vi "GetRadialProfile2.vi"(0 "Which \nRadial Profile? 2":enum16{"Cold Image", "Hot/Cold", "Hot Image"}(ring)=enum."Hot/Cold" caption="Which Radial Profile?", 1 "Paths in Folder":path[](array[path])=[path "C:/Daten/pHGradienten/130403_Cy5_74mer_TRIS/130403_Cy5_74mer_TRIS/A_50mM_TRIS/50mA/TRIS_50mM_50mA_000001.tif", path "C:/Daten/pHGradienten/130403_Cy5_74mer_TRIS/130403_Cy5_74mer_TRIS/A_50mM_TRIS/50mA/TRIS_50mM_50mA_000002.tif", path "C:/Daten/pHGradienten/130403_Cy5_74mer_TRIS/130403_Cy5_74mer_TRIS/A_50mM_TRIS/50mA/TRIS_50mM_50mA_000003.tif", path "C:/Daten/pHGradienten/130403_Cy5_74mer_TRIS/130403_Cy5_74mer_TRIS/A_50mM_TRIS/50mA/TRIS_50mM_50mA_000004.tif", path "C:/Daten/pHGradienten/130403_Cy5_74mer_TRIS/130403_Cy5_74mer_TRIS/A_50mM_TRIS/50mA/TRIS_50mM_50mA_000005.tif", path "C:/Daten/pHGradienten/130403_Cy5_74mer_TRIS/130403_Cy5_74mer_TRIS/A_50mM_TRIS/50mA/TRIS_50mM_50mA_000006.tif", path "C:/Daten/pHGradienten/130403_Cy5_74mer_TRIS/130403_Cy5_74mer_TRIS/A_50mM_TRIS/50mA/TRIS_50mM_50mA_000007.tif", path "C:/Daten/pHGradienten/130403_Cy5_74mer_TRIS/130403_Cy5_74mer_TRIS/A_50mM_TRIS/50mA/TRIS_50mM_50mA_000008.tif", path "C:/Daten/pHGradienten/130403_Cy5_74mer_TRIS/130403_Cy5_74mer_TRIS/A_50mM_TRIS/50mA/TRIS_50mM_50mA_000009.tif", path "C:/Daten/pHGradienten/130403_Cy5_74mer_TRIS/130403_Cy5_74mer_TRIS/A_50mM_TRIS/50mA/TRIS_50mM_50mA_000010.tif", path "C:/Daten/pHGradienten/130403_Cy5_74mer_TRIS/130403_Cy5_74mer_TRIS/A_50mM_TRIS/50mA/TRIS_50mM_50mA_000011.tif", path "C:/Daten/pHGradienten/130403_Cy5_74mer_TRIS/130403_Cy5_74mer_TRIS/A_50mM_TRIS/50mA/TRIS_50mM_50mA_000012.tif", path "C:/Daten/pHGradienten/130403_Cy5_74mer_TRIS/130403_Cy5_74mer_TRIS/A_50mM_TRIS/50mA/TRIS_50mM_50mA_000013.tif", path "C:/Daten/pHGradienten/130403_Cy5_74mer_TRIS/130403_Cy5_74mer_TRIS/A_50mM_TRIS/50mA/TRIS_50mM_50mA_000014.tif", path "C:/Daten/pHGradienten/130403_Cy5_74mer_TRIS/130403_Cy5_74mer_TRIS/A_50mM_TRIS/50mA/TRIS_50mM_50mA_000015.tif", path "C:/Daten/pHGradienten/130403_Cy5_74mer_TRIS/130403_Cy5_74mer_TRIS/A_50mM_TRIS/50mA/TRIS_50mM_50mA_000016.tif", path "C:/Daten/pHGradienten/130403_Cy5_74mer_TRIS/130403_Cy5_74mer_TRIS/A_50mM_TRIS/50mA/TRIS_50mM_50mA_000017.tif", path "C:/Daten/pHGradienten/130403_Cy5_74mer_TRIS/130403_Cy5_74mer_TRIS/A_50mM_TRIS/50mA/TRIS_50mM_50mA_000018.tif", path "C:/Daten/pHGradienten/130403_Cy5_74mer_TRIS/130403_Cy5_74mer_TRIS/A_50mM_TRIS/50mA/TRIS_50mM_50mA_000019.tif", path "C:/Daten/pHGradienten/130403_Cy5_74mer_TRIS/130403_Cy5_74mer_TRIS/A_50mM_TRIS/50mA/TRIS_50mM_50mA_000020.tif", path "C:/Daten/pHGradienten/130403_Cy5_74mer_TRIS/130403_Cy5_74mer_TRIS/A_50mM_TRIS/50mA/TRIS_50mM_50mA_000021.tif", path "C:/Daten/pHGradienten/130403_Cy5_74mer_TRIS/130403_Cy5_74mer_TRIS/A_50mM_TRIS/50mA/TRIS_50mM_50mA_000022.tif", path "C:/Daten/pHGradienten/130403_Cy5_74mer_TRIS/130403_Cy5_74mer_TRIS/A_50mM_TRIS/50mA/TRIS_50mM_50mA_000023.tif", path "C:/Daten/pHGradienten/130403_Cy5_74mer_TRIS/130403_Cy5_74mer_TRIS/A_50mM_TRIS/50mA/TRIS_50mM_50mA_000024.tif", path "C:/Daten/pHGradienten/130403_Cy5_74mer_TRIS/130403_Cy5_74mer_TRIS/A_50mM_TRIS/50mA/TRIS_50mM_50mA_000025.tif", path "C:/Daten/pHGradienten/130403_Cy5_74mer_TRIS/130403_Cy5_74mer_TRIS/A_50mM_TRIS/50mA/TRIS_50mM_50mA_000026.tif", path "C:/Daten/pHGradienten/130403_Cy5_74mer_TRIS/130403_Cy5_74mer_TRIS/A_50mM_TRIS/50mA/TRIS_50mM_50mA_000027.tif", path "C:/Daten/pHGradienten/130403_Cy5_74mer_TRIS/130403_Cy5_74mer_TRIS/A_50mM_TRIS/50mA/TRIS_50mM_50mA_000028.tif", path "C:/Daten/pHGradienten/130403_Cy5_74mer_TRIS/130403_Cy5_74mer_TRIS/A_50mM_TRIS/50mA/TRIS_50mM_50mA_000029.tif", path "C:/Daten/pHGradienten/130403_Cy5_74mer_TRIS/130403_Cy5_74mer_TRIS/A_50mM_TRIS/50mA/TRIS_50mM_50mA_000030.tif", path "C:/Daten/pHGradienten/130403_Cy5_74mer_TRIS/130403_Cy5_74mer_TRIS/A_50mM_TRIS/50mA/TRIS_50mM_50mA_000031.tif", path "C:/Daten/pHGradienten/130403_Cy5_74mer_TRIS/130403_Cy5_74mer_TRIS/A_50mM_TRIS/50mA/TRIS_50mM_50mA_000032.tif", path "C:/Daten/pHGradienten/130403_Cy5_74mer_TRIS/130403_Cy5_74mer_TRIS/A_50mM_TRIS/50mA/TRIS_50mM_50mA_000033.tif", path "C:/Daten/pHGradienten/130403_Cy5_74mer_TRIS/130403_Cy5_74mer_TRIS/A_50mM_TRIS/50mA/TRIS_50mM_50mA_000034.tif", path "C:/Daten/pHGradienten/130403_Cy5_74mer_TRIS/130403_Cy5_74mer_TRIS/A_50mM_TRIS/50mA/TRIS_50mM_50mA_000035.tif", path "C:/Daten/pHGradienten/130403_Cy5_74mer_TRIS/130403_Cy5_74mer_TRIS/A_50mM_TRIS/50mA/TRIS_50mM_50mA_000036.tif", path "C:/Daten/pHGradienten/130403_Cy5_74mer_TRIS/130403_Cy5_74mer_TRIS/A_50mM_TRIS/50mA/TRIS_50mM_50mA_000037.tif", path "C:/Daten/pHGradienten/130403_Cy5_74mer_TRIS/130403_Cy5_74mer_TRIS/A_50mM_TRIS/50mA/TRIS_50mM_50mA_000038.tif", path "C:/Daten/pHGradienten/130403_Cy5_74mer_TRIS/130403_Cy5_74mer_TRIS/A_50mM_TRIS/50mA/TRIS_50mM_50mA_000039.tif", path "C:/Daten/pHGradienten/130403_Cy5_74mer_TRIS/130403_Cy5_74mer_TRIS/A_50mM_TRIS/50mA/TRIS_50mM_50mA_000040.tif", path "C:/Daten/pHGradienten/130403_Cy5_74mer_TRIS/130403_Cy5_74mer_TRIS/A_50mM_TRIS/50mA/TRIS_50mM_50mA_000041.tif", path "C:/Daten/pHGradienten/130403_Cy5_74mer_TRIS/130403_Cy5_74mer_TRIS/A_50mM_TRIS/50mA/TRIS_50mM_50mA_000042.tif", path "C:/Daten/pHGradienten/130403_Cy5_74mer_TRIS/130403_Cy5_74mer_TRIS/A_50mM_TRIS/50mA/TRIS_50mM_50mA_000043.tif", path "C:/Daten/pHGradienten/130403_Cy5_74mer_TRIS/130403_Cy5_74mer_TRIS/A_50mM_TRIS/50mA/TRIS_50mM_50mA_000044.tif", path "C:/Daten/pHGradienten/130403_Cy5_74mer_TRIS/130403_Cy5_74mer_TRIS/A_50mM_TRIS/50mA/TRIS_50mM_50mA_000045.tif", path "C:/Daten/pHGradienten/130403_Cy5_74mer_TRIS/130403_Cy5_74mer_TRIS/A_50mM_TRIS/50mA/TRIS_50mM_50mA_000046.tif", path "C:/Daten/pHGradienten/130403_Cy5_74mer_TRIS/130403_Cy5_74mer_TRIS/A_50mM_TRIS/50mA/TRIS_50mM_50mA_000047.tif", path "C:/Daten/pHGradienten/130403_Cy5_74mer_TRIS/130403_Cy5_74mer_TRIS/A_50mM_TRIS/50mA/TRIS_50mM_50mA_000048.tif", path "C:/Daten/pHGradienten/130403_Cy5_74mer_TRIS/130403_Cy5_74mer_TRIS/A_50mM_TRIS/50mA/TRIS_50mM_50mA_000049.tif", path "C:/Daten/pHGradienten/130403_Cy5_74mer_TRIS/130403_Cy5_74mer_TRIS/A_50mM_TRIS/50mA/TRIS_50mM_50mA_000050.tif", path "C:/Daten/pHGradienten/130403_Cy5_74mer_TRIS/130403_Cy5_74mer_TRIS/A_50mM_TRIS/50mA/TRIS_50mM_50mA_000051.tif", path "C:/Daten/pHGradienten/130403_Cy5_74mer_TRIS/130403_Cy5_74mer_TRIS/A_50mM_TRIS/50mA/TRIS_50mM_50mA_000052.tif", path "C:/Daten/pHGradienten/130403_Cy5_74mer_TRIS/130403_Cy5_74mer_TRIS/A_50mM_TRIS/50mA/TRIS_50mM_50mA_000053.tif", path "C:/Daten/pHGradienten/130403_Cy5_74mer_TRIS/130403_Cy5_74mer_TRIS/A_50mM_TRIS/50mA/TRIS_50mM_50mA_000054.tif", path "C:/Daten/pHGradienten/130403_Cy5_74mer_TRIS/130403_Cy5_74mer_TRIS/A_50mM_TRIS/50mA/TRIS_50mM_50mA_000055.tif", path "C:/Daten/pHGradienten/130403_Cy5_74mer_TRIS/130403_Cy5_74mer_TRIS/A_50mM_TRIS/50mA/TRIS_50mM_50mA_000056.tif", path "C:/Daten/pHGradienten/130403_Cy5_74mer_TRIS/130403_Cy5_74mer_TRIS/A_50mM_TRIS/50mA/TRIS_50mM_50mA_000057.tif", path "C:/Daten/pHGradienten/130403_Cy5_74mer_TRIS/130403_Cy5_74mer_TRIS/A_50mM_TRIS/50mA/TRIS_50mM_50mA_000058.tif", path "C:/Daten/pHGradienten/130403_Cy5_74mer_TRIS/130403_Cy5_74mer_TRIS/A_50mM_TRIS/50mA/TRIS_50mM_50mA_000059.tif", path "C:/Daten/pHGradienten/130403_Cy5_74mer_TRIS/130403_Cy5_74mer_TRIS/A_50mM_TRIS/50mA/TRIS_50mM_50mA_000060.tif", path "C:/Daten/pHGradienten/130403_Cy5_74mer_TRIS/130403_Cy5_74mer_TRIS/A_50mM_TRIS/50mA/TRIS_50mM_50mA_000061.tif", path "C:/Daten/pHGradienten/130403_Cy5_74mer_TRIS/130403_Cy5_74mer_TRIS/A_50mM_TRIS/50mA/TRIS_50mM_50mA_000062.tif", path "C:/Daten/pHGradienten/130403_Cy5_74mer_TRIS/130403_Cy5_74mer_TRIS/A_50mM_TRIS/50mA/TRIS_50mM_50mA_000063.tif", path "C:/Daten/pHGradienten/130403_Cy5_74mer_TRIS/130403_Cy5_74mer_TRIS/A_50mM_TRIS/50mA/TRIS_50mM_50mA_000064.tif", path "C:/Daten/pHGradienten/130403_Cy5_74mer_TRIS/130403_Cy5_74mer_TRIS/A_50mM_TRIS/50mA/TRIS_50mM_50mA_000065.tif", path "C:/Daten/pHGradienten/130403_Cy5_74mer_TRIS/130403_Cy5_74mer_TRIS/A_50mM_TRIS/50mA/TRIS_50mM_50mA_000066.tif", path "C:/Daten/pHGradienten/130403_Cy5_74mer_TRIS/130403_Cy5_74mer_TRIS/A_50mM_TRIS/50mA/TRIS_50mM_50mA_000067.tif", path "C:/Daten/pHGradienten/130403_Cy5_74mer_TRIS/130403_Cy5_74mer_TRIS/A_50mM_TRIS/50mA/TRIS_50mM_50mA_000068.tif", path "C:/Daten/pHGradienten/130403_Cy5_74mer_TRIS/130403_Cy5_74mer_TRIS/A_50mM_TRIS/50mA/TRIS_50mM_50mA_000069.tif", path "C:/Daten/pHGradienten/130403_Cy5_74mer_TRIS/130403_Cy5_74mer_TRIS/A_50mM_TRIS/50mA/TRIS_50mM_50mA_000070.tif", path "C:/Daten/pHGradienten/130403_Cy5_74mer_TRIS/130403_Cy5_74mer_TRIS/A_50mM_TRIS/50mA/TRIS_50mM_50mA_000071.tif", path "C:/Daten/pHGradienten/130403_Cy5_74mer_TRIS/130403_Cy5_74mer_TRIS/A_50mM_TRIS/50mA/TRIS_50mM_50mA_000072.tif", path "C:/Daten/pHGradienten/130403_Cy5_74mer_TRIS/130403_Cy5_74mer_TRIS/A_50mM_TRIS/50mA/TRIS_50mM_50mA_000073.tif", path "C:/Daten/pHGradienten/130403_Cy5_74mer_TRIS/130403_Cy5_74mer_TRIS/A_50mM_TRIS/50mA/TRIS_50mM_50mA_000074.tif", path "C:/Daten/pHGradienten/130403_Cy5_74mer_TRIS/130403_Cy5_74mer_TRIS/A_50mM_TRIS/50mA/TRIS_50mM_50mA_000075.tif", path "C:/Daten/pHGradienten/130403_Cy5_74mer_TRIS/130403_Cy5_74mer_TRIS/A_50mM_TRIS/50mA/TRIS_50mM_50mA_000076.tif", path "C:/Daten/pHGradienten/130403_Cy5_74mer_TRIS/130403_Cy5_74mer_TRIS/A_50mM_TRIS/50mA/TRIS_50mM_50mA_000077.tif", path "C:/Daten/pHGradienten/130403_Cy5_74mer_TRIS/130403_Cy5_74mer_TRIS/A_50mM_TRIS/50mA/TRIS_50mM_50mA_000078.tif", path "C:/Daten/pHGradienten/130403_Cy5_74mer_TRIS/130403_Cy5_74mer_TRIS/A_50mM_TRIS/50mA/TRIS_50mM_50mA_000079.tif", path "C:/Daten/pHGradienten/130403_Cy5_74mer_TRIS/130403_Cy5_74mer_TRIS/A_50mM_TRIS/50mA/TRIS_50mM_50mA_000080.tif", path "C:/Daten/pHGradienten/130403_Cy5_74mer_TRIS/130403_Cy5_74mer_TRIS/A_50mM_TRIS/50mA/TRIS_50mM_50mA_000081.tif", path "C:/Daten/pHGradienten/130403_Cy5_74mer_TRIS/130403_Cy5_74mer_TRIS/A_50mM_TRIS/50mA/TRIS_50mM_50mA_000082.tif", path "C:/Daten/pHGradienten/130403_Cy5_74mer_TRIS/130403_Cy5_74mer_TRIS/A_50mM_TRIS/50mA/TRIS_50mM_50mA_000083.tif", path "C:/Daten/pHGradienten/130403_Cy5_74mer_TRIS/130403_Cy5_74mer_TRIS/A_50mM_TRIS/50mA/TRIS_50mM_50mA_000084.tif", path "C:/Daten/pHGradienten/130403_Cy5_74mer_TRIS/130403_Cy5_74mer_TRIS/A_50mM_TRIS/50mA/TRIS_50mM_50mA_000085.tif", path "C:/Daten/pHGradienten/130403_Cy5_74mer_TRIS/130403_Cy5_74mer_TRIS/A_50mM_TRIS/50mA/TRIS_50mM_50mA_000086.tif", path "C:/Daten/pHGradienten/130403_Cy5_74mer_TRIS/130403_Cy5_74mer_TRIS/A_50mM_TRIS/50mA/TRIS_50mM_50mA_000087.tif", path "C:/Daten/pHGradienten/130403_Cy5_74mer_TRIS/130403_Cy5_74mer_TRIS/A_50mM_TRIS/50mA/TRIS_50mM_50mA_000088.tif", path "C:/Daten/pHGradienten/130403_Cy5_74mer_TRIS/130403_Cy5_74mer_TRIS/A_50mM_TRIS/50mA/TRIS_50mM_50mA_000089.tif", path "C:/Daten/pHGradienten/130403_Cy5_74mer_TRIS/130403_Cy5_74mer_TRIS/A_50mM_TRIS/50mA/TRIS_50mM_50mA_000090.tif", path "C:/Daten/pHGradienten/130403_Cy5_74mer_TRIS/130403_Cy5_74mer_TRIS/A_50mM_TRIS/50mA/TRIS_50mM_50mA_000091.tif", path "C:/Daten/pHGradienten/130403_Cy5_74mer_TRIS/130403_Cy5_74mer_TRIS/A_50mM_TRIS/50mA/TRIS_50mM_50mA_000092.tif", path "C:/Daten/pHGradienten/130403_Cy5_74mer_TRIS/130403_Cy5_74mer_TRIS/A_50mM_TRIS/50mA/TRIS_50mM_50mA_000093.tif", path "C:/Daten/pHGradienten/130403_Cy5_74mer_TRIS/130403_Cy5_74mer_TRIS/A_50mM_TRIS/50mA/TRIS_50mM_50mA_000094.tif", path "C:/Daten/pHGradienten/130403_Cy5_74mer_TRIS/130403_Cy5_74mer_TRIS/A_50mM_TRIS/50mA/TRIS_50mM_50mA_000095.tif", path "C:/Daten/pHGradienten/130403_Cy5_74mer_TRIS/130403_Cy5_74mer_TRIS/A_50mM_TRIS/50mA/TRIS_50mM_50mA_000096.tif", path "C:/Daten/pHGradienten/130403_Cy5_74mer_TRIS/130403_Cy5_74mer_TRIS/A_50mM_TRIS/50mA/TRIS_50mM_50mA_000097.tif", path "C:/Daten/pHGradienten/130403_Cy5_74mer_TRIS/130403_Cy5_74mer_TRIS/A_50mM_TRIS/50mA/TRIS_50mM_50mA_000098.tif", path "C:/Daten/pHGradienten/130403_Cy5_74mer_TRIS/130403_Cy5_74mer_TRIS/A_50mM_TRIS/50mA/TRIS_50mM_50mA_000099.tif", path "C:/Daten/pHGradienten/130403_Cy5_74mer_TRIS/130403_Cy5_74mer_TRIS/A_50mM_TRIS/50mA/TRIS_50mM_50mA_000100.tif", path "C:/Daten/pHGradienten/130403_Cy5_74mer_TRIS/130403_Cy5_74mer_TRIS/A_50mM_TRIS/50mA/TRIS_50mM_50mA_000101.tif", path "C:/Daten/pHGradienten/130403_Cy5_74mer_TRIS/130403_Cy5_74mer_TRIS/A_50mM_TRIS/50mA/TRIS_50mM_50mA_000102.tif", path "C:/Daten/pHGradienten/130403_Cy5_74mer_TRIS/130403_Cy5_74mer_TRIS/A_50mM_TRIS/50mA/TRIS_50mM_50mA_000103.tif", path "C:/Daten/pHGradienten/130403_Cy5_74mer_TRIS/130403_Cy5_74mer_TRIS/A_50mM_TRIS/50mA/TRIS_50mM_50mA_000104.tif", path "C:/Daten/pHGradienten/130403_Cy5_74mer_TRIS/130403_Cy5_74mer_TRIS/A_50mM_TRIS/50mA/TRIS_50mM_50mA_000105.tif", path "C:/Daten/pHGradienten/130403_Cy5_74mer_TRIS/130403_Cy5_74mer_TRIS/A_50mM_TRIS/50mA/TRIS_50mM_50mA_000106.tif", path "C:/Daten/pHGradienten/130403_Cy5_74mer_TRIS/130403_Cy5_74mer_TRIS/A_50mM_TRIS/50mA/TRIS_50mM_50mA_000107.tif", path "C:/Daten/pHGradienten/130403_Cy5_74mer_TRIS/130403_Cy5_74mer_TRIS/A_50mM_TRIS/50mA/TRIS_50mM_50mA_000108.tif", path "C:/Daten/pHGradienten/130403_Cy5_74mer_TRIS/130403_Cy5_74mer_TRIS/A_50mM_TRIS/50mA/TRIS_50mM_50mA_000109.tif", path "C:/Daten/pHGradienten/130403_Cy5_74mer_TRIS/130403_Cy5_74mer_TRIS/A_50mM_TRIS/50mA/TRIS_50mM_50mA_000110.tif", path "C:/Daten/pHGradienten/130403_Cy5_74mer_TRIS/130403_Cy5_74mer_TRIS/A_50mM_TRIS/50mA/TRIS_50mM_50mA_000111.tif", path "C:/Daten/pHGradienten/130403_Cy5_74mer_TRIS/130403_Cy5_74mer_TRIS/A_50mM_TRIS/50mA/TRIS_50mM_50mA_000112.tif", path "C:/Daten/pHGradienten/130403_Cy5_74mer_TRIS/130403_Cy5_74mer_TRIS/A_50mM_TRIS/50mA/TRIS_50mM_50mA_000113.tif", path "C:/Daten/pHGradienten/130403_Cy5_74mer_TRIS/130403_Cy5_74mer_TRIS/A_50mM_TRIS/50mA/TRIS_50mM_50mA_000114.tif", path "C:/Daten/pHGradienten/130403_Cy5_74mer_TRIS/130403_Cy5_74mer_TRIS/A_50mM_TRIS/50mA/TRIS_50mM_50mA_000115.tif", path "C:/Daten/pHGradienten/130403_Cy5_74mer_TRIS/130403_Cy5_74mer_TRIS/A_50mM_TRIS/50mA/TRIS_50mM_50mA_000116.tif", path "C:/Daten/pHGradienten/130403_Cy5_74mer_TRIS/130403_Cy5_74mer_TRIS/A_50mM_TRIS/50mA/TRIS_50mM_50mA_000117.tif", path "C:/Daten/pHGradienten/130403_Cy5_74mer_TRIS/130403_Cy5_74mer_TRIS/A_50mM_TRIS/50mA/TRIS_50mM_50mA_000118.tif", path "C:/Daten/pHGradienten/130403_Cy5_74mer_TRIS/130403_Cy5_74mer_TRIS/A_50mM_TRIS/50mA/TRIS_50mM_50mA_000119.tif", path "C:/Daten/pHGradienten/130403_Cy5_74mer_TRIS/130403_Cy5_74mer_TRIS/A_50mM_TRIS/50mA/TRIS_50mM_50mA_000120.tif", path "C:/Daten/pHGradienten/130403_Cy5_74mer_TRIS/130403_Cy5_74mer_TRIS/A_50mM_TRIS/50mA/TRIS_50mM_50mA_000121.tif", path "C:/Daten/pHGradienten/130403_Cy5_74mer_TRIS/130403_Cy5_74mer_TRIS/A_50mM_TRIS/50mA/TRIS_50mM_50mA_000122.tif", path "C:/Daten/pHGradienten/130403_Cy5_74mer_TRIS/130403_Cy5_74mer_TRIS/A_50mM_TRIS/50mA/TRIS_50mM_50mA_000123.tif", path "C:/Daten/pHGradienten/130403_Cy5_74mer_TRIS/130403_Cy5_74mer_TRIS/A_50mM_TRIS/50mA/TRIS_50mM_50mA_000124.tif", path "C:/Daten/pHGradienten/130403_Cy5_74mer_TRIS/130403_Cy5_74mer_TRIS/A_50mM_TRIS/50mA/TRIS_50mM_50mA_000125.tif", path "C:/Daten/pHGradienten/130403_Cy5_74mer_TRIS/130403_Cy5_74mer_TRIS/A_50mM_TRIS/50mA/TRIS_50mM_50mA_000126.tif", path "C:/Daten/pHGradienten/130403_Cy5_74mer_TRIS/130403_Cy5_74mer_TRIS/A_50mM_TRIS/50mA/TRIS_50mM_50mA_000127.tif", path "C:/Daten/pHGradienten/130403_Cy5_74mer_TRIS/130403_Cy5_74mer_TRIS/A_50mM_TRIS/50mA/TRIS_50mM_50mA_000128.tif", path "C:/Daten/pHGradienten/130403_Cy5_74mer_TRIS/130403_Cy5_74mer_TRIS/A_50mM_TRIS/50mA/TRIS_50mM_50mA_000129.tif", path "C:/Daten/pHGradienten/130403_Cy5_74mer_TRIS/130403_Cy5_74mer_TRIS/A_50mM_TRIS/50mA/TRIS_50mM_50mA_000130.tif", path "C:/Daten/pHGradienten/130403_Cy5_74mer_TRIS/130403_Cy5_74mer_TRIS/A_50mM_TRIS/50mA/TRIS_50mM_50mA_000131.tif", path "C:/Daten/pHGradienten/130403_Cy5_74mer_TRIS/130403_Cy5_74mer_TRIS/A_50mM_TRIS/50mA/TRIS_50mM_50mA_000132.tif", path "C:/Daten/pHGradienten/130403_Cy5_74mer_TRIS/130403_Cy5_74mer_TRIS/A_50mM_TRIS/50mA/TRIS_50mM_50mA_000133.tif", path "C:/Daten/pHGradienten/130403_Cy5_74mer_TRIS/130403_Cy5_74mer_TRIS/A_50mM_TRIS/50mA/TRIS_50mM_50mA_000134.tif", path "C:/Daten/pHGradienten/130403_Cy5_74mer_TRIS/130403_Cy5_74mer_TRIS/A_50mM_TRIS/50mA/TRIS_50mM_50mA_000135.tif", path "C:/Daten/pHGradienten/130403_Cy5_74mer_TRIS/130403_Cy5_74mer_TRIS/A_50mM_TRIS/50mA/TRIS_50mM_50mA_000136.tif", path "C:/Daten/pHGradienten/130403_Cy5_74mer_TRIS/130403_Cy5_74mer_TRIS/A_50mM_TRIS/50mA/TRIS_50mM_50mA_000137.tif", path "C:/Daten/pHGradienten/130403_Cy5_74mer_TRIS/130403_Cy5_74mer_TRIS/A_50mM_TRIS/50mA/TRIS_50mM_50mA_000138.tif", path "C:/Daten/pHGradienten/130403_Cy5_74mer_TRIS/130403_Cy5_74mer_TRIS/A_50mM_TRIS/50mA/TRIS_50mM_50mA_000139.tif", path "C:/Daten/pHGradienten/130403_Cy5_74mer_TRIS/130403_Cy5_74mer_TRIS/A_50mM_TRIS/50mA/TRIS_50mM_50mA_000140.tif", path "C:/Daten/pHGradienten/130403_Cy5_74mer_TRIS/130403_Cy5_74mer_TRIS/A_50mM_TRIS/50mA/TRIS_50mM_50mA_000141.tif", path "C:/Daten/pHGradienten/130403_Cy5_74mer_TRIS/130403_Cy5_74mer_TRIS/A_50mM_TRIS/50mA/TRIS_50mM_50mA_000142.tif", path "C:/Daten/pHGradienten/130403_Cy5_74mer_TRIS/130403_Cy5_74mer_TRIS/A_50mM_TRIS/50mA/TRIS_50mM_50mA_000143.tif", path "C:/Daten/pHGradienten/130403_Cy5_74mer_TRIS/130403_Cy5_74mer_TRIS/A_50mM_TRIS/50mA/TRIS_50mM_50mA_000144.tif", path "C:/Daten/pHGradienten/130403_Cy5_74mer_TRIS/130403_Cy5_74mer_TRIS/A_50mM_TRIS/50mA/TRIS_50mM_50mA_000145.tif", path "C:/Daten/pHGradienten/130403_Cy5_74mer_TRIS/130403_Cy5_74mer_TRIS/A_50mM_TRIS/50mA/TRIS_50mM_50mA_000146.tif", path "C:/Daten/pHGradienten/130403_Cy5_74mer_TRIS/130403_Cy5_74mer_TRIS/A_50mM_TRIS/50mA/TRIS_50mM_50mA_000147.tif", path "C:/Daten/pHGradienten/130403_Cy5_74mer_TRIS/130403_Cy5_74mer_TRIS/A_50mM_TRIS/50mA/TRIS_50mM_50mA_000148.tif", path "C:/Daten/pHGradienten/130403_Cy5_74mer_TRIS/130403_Cy5_74mer_TRIS/A_50mM_TRIS/50mA/TRIS_50mM_50mA_000149.tif", path "C:/Daten/pHGradienten/130403_Cy5_74mer_TRIS/130403_Cy5_74mer_TRIS/A_50mM_TRIS/50mA/TRIS_50mM_50mA_000150.tif", path "C:/Daten/pHGradienten/130403_Cy5_74mer_TRIS/130403_Cy5_74mer_TRIS/A_50mM_TRIS/50mA/TRIS_50mM_50mA_000151.tif", path "C:/Daten/pHGradienten/130403_Cy5_74mer_TRIS/130403_Cy5_74mer_TRIS/A_50mM_TRIS/50mA/TRIS_50mM_50mA_000152.tif", path "C:/Daten/pHGradienten/130403_Cy5_74mer_TRIS/130403_Cy5_74mer_TRIS/A_50mM_TRIS/50mA/TRIS_50mM_50mA_000153.tif", path "C:/Daten/pHGradienten/130403_Cy5_74mer_TRIS/130403_Cy5_74mer_TRIS/A_50mM_TRIS/50mA/TRIS_50mM_50mA_000154.tif", path "C:/Daten/pHGradienten/130403_Cy5_74mer_TRIS/130403_Cy5_74mer_TRIS/A_50mM_TRIS/50mA/TRIS_50mM_50mA_000155.tif", path "C:/Daten/pHGradienten/130403_Cy5_74mer_TRIS/130403_Cy5_74mer_TRIS/A_50mM_TRIS/50mA/TRIS_50mM_50mA_000156.tif", path "C:/Daten/pHGradienten/130403_Cy5_74mer_TRIS/130403_Cy5_74mer_TRIS/A_50mM_TRIS/50mA/TRIS_50mM_50mA_000157.tif", path "C:/Daten/pHGradienten/130403_Cy5_74mer_TRIS/130403_Cy5_74mer_TRIS/A_50mM_TRIS/50mA/TRIS_50mM_50mA_000158.tif", path "C:/Daten/pHGradienten/130403_Cy5_74mer_TRIS/130403_Cy5_74mer_TRIS/A_50mM_TRIS/50mA/TRIS_50mM_50mA_000159.tif", path "C:/Daten/pHGradienten/130403_Cy5_74mer_TRIS/130403_Cy5_74mer_TRIS/A_50mM_TRIS/50mA/TRIS_50mM_50mA_000160.tif", path "C:/Daten/pHGradienten/130403_Cy5_74mer_TRIS/130403_Cy5_74mer_TRIS/A_50mM_TRIS/50mA/TRIS_50mM_50mA_000161.tif", path "C:/Daten/pHGradienten/130403_Cy5_74mer_TRIS/130403_Cy5_74mer_TRIS/A_50mM_TRIS/50mA/TRIS_50mM_50mA_000162.tif", path "C:/Daten/pHGradienten/130403_Cy5_74mer_TRIS/130403_Cy5_74mer_TRIS/A_50mM_TRIS/50mA/TRIS_50mM_50mA_000163.tif", path "C:/Daten/pHGradienten/130403_Cy5_74mer_TRIS/130403_Cy5_74mer_TRIS/A_50mM_TRIS/50mA/TRIS_50mM_50mA_000164.tif", path "C:/Daten/pHGradienten/130403_Cy5_74mer_TRIS/130403_Cy5_74mer_TRIS/A_50mM_TRIS/50mA/TRIS_50mM_50mA_000165.tif", path "C:/Daten/pHGradienten/130403_Cy5_74mer_TRIS/130403_Cy5_74mer_TRIS/A_50mM_TRIS/50mA/TRIS_50mM_50mA_000166.tif", path "C:/Daten/pHGradienten/130403_Cy5_74mer_TRIS/130403_Cy5_74mer_TRIS/A_50mM_TRIS/50mA/TRIS_50mM_50mA_000167.tif", path "C:/Daten/pHGradienten/130403_Cy5_74mer_TRIS/130403_Cy5_74mer_TRIS/A_50mM_TRIS/50mA/TRIS_50mM_50mA_000168.tif", path "C:/Daten/pHGradienten/130403_Cy5_74mer_TRIS/130403_Cy5_74mer_TRIS/A_50mM_TRIS/50mA/TRIS_50mM_50mA_000169.tif", path "C:/Daten/pHGradienten/130403_Cy5_74mer_TRIS/130403_Cy5_74mer_TRIS/A_50mM_TRIS/50mA/TRIS_50mM_50mA_000170.tif", path "C:/Daten/pHGradienten/130403_Cy5_74mer_TRIS/130403_Cy5_74mer_TRIS/A_50mM_TRIS/50mA/TRIS_50mM_50mA_000171.tif", path "C:/Daten/pHGradienten/130403_Cy5_74mer_TRIS/130403_Cy5_74mer_TRIS/A_50mM_TRIS/50mA/TRIS_50mM_50mA_000172.tif", path "C:/Daten/pHGradienten/130403_Cy5_74mer_TRIS/130403_Cy5_74mer_TRIS/A_50mM_TRIS/50mA/TRIS_50mM_50mA_000173.tif", path "C:/Daten/pHGradienten/130403_Cy5_74mer_TRIS/130403_Cy5_74mer_TRIS/A_50mM_TRIS/50mA/TRIS_50mM_50mA_000174.tif", path "C:/Daten/pHGradienten/130403_Cy5_74mer_TRIS/130403_Cy5_74mer_TRIS/A_50mM_TRIS/50mA/TRIS_50mM_50mA_000175.tif", path "C:/Daten/pHGradienten/130403_Cy5_74mer_TRIS/130403_Cy5_74mer_TRIS/A_50mM_TRIS/50mA/TRIS_50mM_50mA_000176.tif", path "C:/Daten/pHGradienten/130403_Cy5_74mer_TRIS/130403_Cy5_74mer_TRIS/A_50mM_TRIS/50mA/TRIS_50mM_50mA_000177.tif", path "C:/Daten/pHGradienten/130403_Cy5_74mer_TRIS/130403_Cy5_74mer_TRIS/A_50mM_TRIS/50mA/TRIS_50mM_50mA_000178.tif", path "C:/Daten/pHGradienten/130403_Cy5_74mer_TRIS/130403_Cy5_74mer_TRIS/A_50mM_TRIS/50mA/TRIS_50mM_50mA_000179.tif", path "C:/Daten/pHGradienten/130403_Cy5_74mer_TRIS/130403_Cy5_74mer_TRIS/A_50mM_TRIS/50mA/TRIS_50mM_50mA_000180.tif", path "C:/Daten/pHGradienten/130403_Cy5_74mer_TRIS/130403_Cy5_74mer_TRIS/A_50mM_TRIS/50mA/TRIS_50mM_50mA_000181.tif", path "C:/Daten/pHGradienten/130403_Cy5_74mer_TRIS/130403_Cy5_74mer_TRIS/A_50mM_TRIS/50mA/TRIS_50mM_50mA_000182.tif", path "C:/Daten/pHGradienten/130403_Cy5_74mer_TRIS/130403_Cy5_74mer_TRIS/A_50mM_TRIS/50mA/TRIS_50mM_50mA_000183.tif", path "C:/Daten/pHGradienten/130403_Cy5_74mer_TRIS/130403_Cy5_74mer_TRIS/A_50mM_TRIS/50mA/TRIS_50mM_50mA_000184.tif", path "C:/Daten/pHGradienten/130403_Cy5_74mer_TRIS/130403_Cy5_74mer_TRIS/A_50mM_TRIS/50mA/TRIS_50mM_50mA_000185.tif", path "C:/Daten/pHGradienten/130403_Cy5_74mer_TRIS/130403_Cy5_74mer_TRIS/A_50mM_TRIS/50mA/TRIS_50mM_50mA_000186.tif", path "C:/Daten/pHGradienten/130403_Cy5_74mer_TRIS/130403_Cy5_74mer_TRIS/A_50mM_TRIS/50mA/TRIS_50mM_50mA_000187.tif", path "C:/Daten/pHGradienten/130403_Cy5_74mer_TRIS/130403_Cy5_74mer_TRIS/A_50mM_TRIS/50mA/TRIS_50mM_50mA_000188.tif", path "C:/Daten/pHGradienten/130403_Cy5_74mer_TRIS/130403_Cy5_74mer_TRIS/A_50mM_TRIS/50mA/TRIS_50mM_50mA_000189.tif", path "C:/Daten/pHGradienten/130403_Cy5_74mer_TRIS/130403_Cy5_74mer_TRIS/A_50mM_TRIS/50mA/TRIS_50mM_50mA_000190.tif", path "C:/Daten/pHGradienten/130403_Cy5_74mer_TRIS/130403_Cy5_74mer_TRIS/A_50mM_TRIS/50mA/TRIS_50mM_50mA_000191.tif", path "C:/Daten/pHGradienten/130403_Cy5_74mer_TRIS/130403_Cy5_74mer_TRIS/A_50mM_TRIS/50mA/TRIS_50mM_50mA_000192.tif", path "C:/Daten/pHGradienten/130403_Cy5_74mer_TRIS/130403_Cy5_74mer_TRIS/A_50mM_TRIS/50mA/TRIS_50mM_50mA_000193.tif", path "C:/Daten/pHGradienten/130403_Cy5_74mer_TRIS/130403_Cy5_74mer_TRIS/A_50mM_TRIS/50mA/TRIS_50mM_50mA_000194.tif", path "C:/Daten/pHGradienten/130403_Cy5_74mer_TRIS/130403_Cy5_74mer_TRIS/A_50mM_TRIS/50mA/TRIS_50mM_50mA_000195.tif", path "C:/Daten/pHGradienten/130403_Cy5_74mer_TRIS/130403_Cy5_74mer_TRIS/A_50mM_TRIS/50mA/TRIS_50mM_50mA_000196.tif", path "C:/Daten/pHGradienten/130403_Cy5_74mer_TRIS/130403_Cy5_74mer_TRIS/A_50mM_TRIS/50mA/TRIS_50mM_50mA_000197.tif", path "C:/Daten/pHGradienten/130403_Cy5_74mer_TRIS/130403_Cy5_74mer_TRIS/A_50mM_TRIS/50mA/TRIS_50mM_50mA_000198.tif", path "C:/Daten/pHGradienten/130403_Cy5_74mer_TRIS/130403_Cy5_74mer_TRIS/A_50mM_TRIS/50mA/TRIS_50mM_50mA_000199.tif", path "C:/Daten/pHGradienten/130403_Cy5_74mer_TRIS/130403_Cy5_74mer_TRIS/A_50mM_TRIS/50mA/TRIS_50mM_50mA_000200.tif", path "C:/Daten/pHGradienten/130403_Cy5_74mer_TRIS/130403_Cy5_74mer_TRIS/A_50mM_TRIS/50mA/TRIS_50mM_50mA_000201.tif", path "C:/Daten/pHGradienten/130403_Cy5_74mer_TRIS/130403_Cy5_74mer_TRIS/A_50mM_TRIS/50mA/TRIS_50mM_50mA_000202.tif", path "C:/Daten/pHGradienten/130403_Cy5_74mer_TRIS/130403_Cy5_74mer_TRIS/A_50mM_TRIS/50mA/TRIS_50mM_50mA_000203.tif", path "C:/Daten/pHGradienten/130403_Cy5_74mer_TRIS/130403_Cy5_74mer_TRIS/A_50mM_TRIS/50mA/TRIS_50mM_50mA_000204.tif", path "C:/Daten/pHGradienten/130403_Cy5_74mer_TRIS/130403_Cy5_74mer_TRIS/A_50mM_TRIS/50mA/TRIS_50mM_50mA_000205.tif", path "C:/Daten/pHGradienten/130403_Cy5_74mer_TRIS/130403_Cy5_74mer_TRIS/A_50mM_TRIS/50mA/TRIS_50mM_50mA_000206.tif", path "C:/Daten/pHGradienten/130403_Cy5_74mer_TRIS/130403_Cy5_74mer_TRIS/A_50mM_TRIS/50mA/TRIS_50mM_50mA_000207.tif", path "C:/Daten/pHGradienten/130403_Cy5_74mer_TRIS/130403_Cy5_74mer_TRIS/A_50mM_TRIS/50mA/TRIS_50mM_50mA_000208.tif", path "C:/Daten/pHGradienten/130403_Cy5_74mer_TRIS/130403_Cy5_74mer_TRIS/A_50mM_TRIS/50mA/TRIS_50mM_50mA_000209.tif", path "C:/Daten/pHGradienten/130403_Cy5_74mer_TRIS/130403_Cy5_74mer_TRIS/A_50mM_TRIS/50mA/TRIS_50mM_50mA_000210.tif", path "C:/Daten/pHGradienten/130403_Cy5_74mer_TRIS/130403_Cy5_74mer_TRIS/A_50mM_TRIS/50mA/TRIS_50mM_50mA_000211.tif", path "C:/Daten/pHGradienten/130403_Cy5_74mer_TRIS/130403_Cy5_74mer_TRIS/A_50mM_TRIS/50mA/TRIS_50mM_50mA_000212.tif", path "C:/Daten/pHGradienten/130403_Cy5_74mer_TRIS/130403_Cy5_74mer_TRIS/A_50mM_TRIS/50mA/TRIS_50mM_50mA_000213.tif", path "C:/Daten/pHGradienten/130403_Cy5_74mer_TRIS/130403_Cy5_74mer_TRIS/A_50mM_TRIS/50mA/TRIS_50mM_50mA_000214.tif", path "C:/Daten/pHGradienten/130403_Cy5_74mer_TRIS/130403_Cy5_74mer_TRIS/A_50mM_TRIS/50mA/TRIS_50mM_50mA_000215.tif", path "C:/Daten/pHGradienten/130403_Cy5_74mer_TRIS/130403_Cy5_74mer_TRIS/A_50mM_TRIS/50mA/TRIS_50mM_50mA_000216.tif", path "C:/Daten/pHGradienten/130403_Cy5_74mer_TRIS/130403_Cy5_74mer_TRIS/A_50mM_TRIS/50mA/TRIS_50mM_50mA_000217.tif", path "C:/Daten/pHGradienten/130403_Cy5_74mer_TRIS/130403_Cy5_74mer_TRIS/A_50mM_TRIS/50mA/TRIS_50mM_50mA_000218.tif", path "C:/Daten/pHGradienten/130403_Cy5_74mer_TRIS/130403_Cy5_74mer_TRIS/A_50mM_TRIS/50mA/TRIS_50mM_50mA_000219.tif", path "C:/Daten/pHGradienten/130403_Cy5_74mer_TRIS/130403_Cy5_74mer_TRIS/A_50mM_TRIS/50mA/TRIS_50mM_50mA_000220.tif", path "C:/Daten/pHGradienten/130403_Cy5_74mer_TRIS/130403_Cy5_74mer_TRIS/A_50mM_TRIS/50mA/TRIS_50mM_50mA_000221.tif", path "C:/Daten/pHGradienten/130403_Cy5_74mer_TRIS/130403_Cy5_74mer_TRIS/A_50mM_TRIS/50mA/TRIS_50mM_50mA_000222.tif", path "C:/Daten/pHGradienten/130403_Cy5_74mer_TRIS/130403_Cy5_74mer_TRIS/A_50mM_TRIS/50mA/TRIS_50mM_50mA_000223.tif", path "C:/Daten/pHGradienten/130403_Cy5_74mer_TRIS/130403_Cy5_74mer_TRIS/A_50mM_TRIS/50mA/TRIS_50mM_50mA_000224.tif", path "C:/Daten/pHGradienten/130403_Cy5_74mer_TRIS/130403_Cy5_74mer_TRIS/A_50mM_TRIS/50mA/TRIS_50mM_50mA_000225.tif", path "C:/Daten/pHGradienten/130403_Cy5_74mer_TRIS/130403_Cy5_74mer_TRIS/A_50mM_TRIS/50mA/TRIS_50mM_50mA_000226.tif", path "C:/Daten/pHGradienten/130403_Cy5_74mer_TRIS/130403_Cy5_74mer_TRIS/A_50mM_TRIS/50mA/TRIS_50mM_50mA_000227.tif", path "C:/Daten/pHGradienten/130403_Cy5_74mer_TRIS/130403_Cy5_74mer_TRIS/A_50mM_TRIS/50mA/TRIS_50mM_50mA_000228.tif", path "C:/Daten/pHGradienten/130403_Cy5_74mer_TRIS/130403_Cy5_74mer_TRIS/A_50mM_TRIS/50mA/TRIS_50mM_50mA_000229.tif", path "C:/Daten/pHGradienten/130403_Cy5_74mer_TRIS/130403_Cy5_74mer_TRIS/A_50mM_TRIS/50mA/TRIS_50mM_50mA_000230.tif", path "C:/Daten/pHGradienten/130403_Cy5_74mer_TRIS/130403_Cy5_74mer_TRIS/A_50mM_TRIS/50mA/TRIS_50mM_50mA_000231.tif", path "C:/Daten/pHGradienten/130403_Cy5_74mer_TRIS/130403_Cy5_74mer_TRIS/A_50mM_TRIS/50mA/TRIS_50mM_50mA_000232.tif", path "C:/Daten/pHGradienten/130403_Cy5_74mer_TRIS/130403_Cy5_74mer_TRIS/A_50mM_TRIS/50mA/TRIS_50mM_50mA_000233.tif", path "C:/Daten/pHGradienten/130403_Cy5_74mer_TRIS/130403_Cy5_74mer_TRIS/A_50mM_TRIS/50mA/TRIS_50mM_50mA_000234.tif", path "C:/Daten/pHGradienten/130403_Cy5_74mer_TRIS/130403_Cy5_74mer_TRIS/A_50mM_TRIS/50mA/TRIS_50mM_50mA_000235.tif", path "C:/Daten/pHGradienten/130403_Cy5_74mer_TRIS/130403_Cy5_74mer_TRIS/A_50mM_TRIS/50mA/TRIS_50mM_50mA_000236.tif", path "C:/Daten/pHGradienten/130403_Cy5_74mer_TRIS/130403_Cy5_74mer_TRIS/A_50mM_TRIS/50mA/TRIS_50mM_50mA_000237.tif", path "C:/Daten/pHGradienten/130403_Cy5_74mer_TRIS/130403_Cy5_74mer_TRIS/A_50mM_TRIS/50mA/TRIS_50mM_50mA_000238.tif", path "C:/Daten/pHGradienten/130403_Cy5_74mer_TRIS/130403_Cy5_74mer_TRIS/A_50mM_TRIS/50mA/TRIS_50mM_50mA_000239.tif", path "C:/Daten/pHGradienten/130403_Cy5_74mer_TRIS/130403_Cy5_74mer_TRIS/A_50mM_TRIS/50mA/TRIS_50mM_50mA_000240.tif", path "C:/Daten/pHGradienten/130403_Cy5_74mer_TRIS/130403_Cy5_74mer_TRIS/A_50mM_TRIS/50mA/TRIS_50mM_50mA_000241.tif", path "C:/Daten/pHGradienten/130403_Cy5_74mer_TRIS/130403_Cy5_74mer_TRIS/A_50mM_TRIS/50mA/TRIS_50mM_50mA_000242.tif", path "C:/Daten/pHGradienten/130403_Cy5_74mer_TRIS/130403_Cy5_74mer_TRIS/A_50mM_TRIS/50mA/TRIS_50mM_50mA_000243.tif", path "C:/Daten/pHGradienten/130403_Cy5_74mer_TRIS/130403_Cy5_74mer_TRIS/A_50mM_TRIS/50mA/TRIS_50mM_50mA_000244.tif", path "C:/Daten/pHGradienten/130403_Cy5_74mer_TRIS/130403_Cy5_74mer_TRIS/A_50mM_TRIS/50mA/TRIS_50mM_50mA_000245.tif", path "C:/Daten/pHGradienten/130403_Cy5_74mer_TRIS/130403_Cy5_74mer_TRIS/A_50mM_TRIS/50mA/TRIS_50mM_50mA_000246.tif", path "C:/Daten/pHGradienten/130403_Cy5_74mer_TRIS/130403_Cy5_74mer_TRIS/A_50mM_TRIS/50mA/TRIS_50mM_50mA_000247.tif", path "C:/Daten/pHGradienten/130403_Cy5_74mer_TRIS/130403_Cy5_74mer_TRIS/A_50mM_TRIS/50mA/TRIS_50mM_50mA_000248.tif", path "C:/Daten/pHGradienten/130403_Cy5_74mer_TRIS/130403_Cy5_74mer_TRIS/A_50mM_TRIS/50mA/TRIS_50mM_50mA_000249.tif", path "C:/Daten/pHGradienten/130403_Cy5_74mer_TRIS/130403_Cy5_74mer_TRIS/A_50mM_TRIS/50mA/TRIS_50mM_50mA_000250.tif", path "C:/Daten/pHGradienten/130403_Cy5_74mer_TRIS/130403_Cy5_74mer_TRIS/A_50mM_TRIS/50mA/TRIS_50mM_50mA_000251.tif", path "C:/Daten/pHGradienten/130403_Cy5_74mer_TRIS/130403_Cy5_74mer_TRIS/A_50mM_TRIS/50mA/TRIS_50mM_50mA_000252.tif", path "C:/Daten/pHGradienten/130403_Cy5_74mer_TRIS/130403_Cy5_74mer_TRIS/A_50mM_TRIS/50mA/TRIS_50mM_50mA_000253.tif", path "C:/Daten/pHGradienten/130403_Cy5_74mer_TRIS/130403_Cy5_74mer_TRIS/A_50mM_TRIS/50mA/TRIS_50mM_50mA_000254.tif", path "C:/Daten/pHGradienten/130403_Cy5_74mer_TRIS/130403_Cy5_74mer_TRIS/A_50mM_TRIS/50mA/TRIS_50mM_50mA_000255.tif", path "C:/Daten/pHGradienten/130403_Cy5_74mer_TRIS/130403_Cy5_74mer_TRIS/A_50mM_TRIS/50mA/TRIS_50mM_50mA_000256.tif", path "C:/Daten/pHGradienten/130403_Cy5_74mer_TRIS/130403_Cy5_74mer_TRIS/A_50mM_TRIS/50mA/TRIS_50mM_50mA_000257.tif", path "C:/Daten/pHGradienten/130403_Cy5_74mer_TRIS/130403_Cy5_74mer_TRIS/A_50mM_TRIS/50mA/TRIS_50mM_50mA_000258.tif", path "C:/Daten/pHGradienten/130403_Cy5_74mer_TRIS/130403_Cy5_74mer_TRIS/A_50mM_TRIS/50mA/TRIS_50mM_50mA_000259.tif", path "C:/Daten/pHGradienten/130403_Cy5_74mer_TRIS/130403_Cy5_74mer_TRIS/A_50mM_TRIS/50mA/TRIS_50mM_50mA_000260.tif", path "C:/Daten/pHGradienten/130403_Cy5_74mer_TRIS/130403_Cy5_74mer_TRIS/A_50mM_TRIS/50mA/TRIS_50mM_50mA_000261.tif", path "C:/Daten/pHGradienten/130403_Cy5_74mer_TRIS/130403_Cy5_74mer_TRIS/A_50mM_TRIS/50mA/TRIS_50mM_50mA_000262.tif", path "C:/Daten/pHGradienten/130403_Cy5_74mer_TRIS/130403_Cy5_74mer_TRIS/A_50mM_TRIS/50mA/TRIS_50mM_50mA_000263.tif", path "C:/Daten/pHGradienten/130403_Cy5_74mer_TRIS/130403_Cy5_74mer_TRIS/A_50mM_TRIS/50mA/TRIS_50mM_50mA_000264.tif", path "C:/Daten/pHGradienten/130403_Cy5_74mer_TRIS/130403_Cy5_74mer_TRIS/A_50mM_TRIS/50mA/TRIS_50mM_50mA_000265.tif", path "C:/Daten/pHGradienten/130403_Cy5_74mer_TRIS/130403_Cy5_74mer_TRIS/A_50mM_TRIS/50mA/TRIS_50mM_50mA_000266.tif", path "C:/Daten/pHGradienten/130403_Cy5_74mer_TRIS/130403_Cy5_74mer_TRIS/A_50mM_TRIS/50mA/TRIS_50mM_50mA_000267.tif", path "C:/Daten/pHGradienten/130403_Cy5_74mer_TRIS/130403_Cy5_74mer_TRIS/A_50mM_TRIS/50mA/TRIS_50mM_50mA_000268.tif", path "C:/Daten/pHGradienten/130403_Cy5_74mer_TRIS/130403_Cy5_74mer_TRIS/A_50mM_TRIS/50mA/TRIS_50mM_50mA_000269.tif", path "C:/Daten/pHGradienten/130403_Cy5_74mer_TRIS/130403_Cy5_74mer_TRIS/A_50mM_TRIS/50mA/TRIS_50mM_50mA_000270.tif", path "C:/Daten/pHGradienten/130403_Cy5_74mer_TRIS/130403_Cy5_74mer_TRIS/A_50mM_TRIS/50mA/TRIS_50mM_50mA_000271.tif", path "C:/Daten/pHGradienten/130403_Cy5_74mer_TRIS/130403_Cy5_74mer_TRIS/A_50mM_TRIS/50mA/TRIS_50mM_50mA_000272.tif", path "C:/Daten/pHGradienten/130403_Cy5_74mer_TRIS/130403_Cy5_74mer_TRIS/A_50mM_TRIS/50mA/TRIS_50mM_50mA_000273.tif", path "C:/Daten/pHGradienten/130403_Cy5_74mer_TRIS/130403_Cy5_74mer_TRIS/A_50mM_TRIS/50mA/TRIS_50mM_50mA_000274.tif", path "C:/Daten/pHGradienten/130403_Cy5_74mer_TRIS/130403_Cy5_74mer_TRIS/A_50mM_TRIS/50mA/TRIS_50mM_50mA_000275.tif", path "C:/Daten/pHGradienten/130403_Cy5_74mer_TRIS/130403_Cy5_74mer_TRIS/A_50mM_TRIS/50mA/TRIS_50mM_50mA_000276.tif", path "C:/Daten/pHGradienten/130403_Cy5_74mer_TRIS/130403_Cy5_74mer_TRIS/A_50mM_TRIS/50mA/TRIS_50mM_50mA_000277.tif", path "C:/Daten/pHGradienten/130403_Cy5_74mer_TRIS/130403_Cy5_74mer_TRIS/A_50mM_TRIS/50mA/TRIS_50mM_50mA_000278.tif", path "C:/Daten/pHGradienten/130403_Cy5_74mer_TRIS/130403_Cy5_74mer_TRIS/A_50mM_TRIS/50mA/TRIS_50mM_50mA_000279.tif", path "C:/Daten/pHGradienten/130403_Cy5_74mer_TRIS/130403_Cy5_74mer_TRIS/A_50mM_TRIS/50mA/TRIS_50mM_50mA_000280.tif", path "C:/Daten/pHGradienten/130403_Cy5_74mer_TRIS/130403_Cy5_74mer_TRIS/A_50mM_TRIS/50mA/TRIS_50mM_50mA_000281.tif", path "C:/Daten/pHGradienten/130403_Cy5_74mer_TRIS/130403_Cy5_74mer_TRIS/A_50mM_TRIS/50mA/TRIS_50mM_50mA_000282.tif", path "C:/Daten/pHGradienten/130403_Cy5_74mer_TRIS/130403_Cy5_74mer_TRIS/A_50mM_TRIS/50mA/TRIS_50mM_50mA_000283.tif", path "C:/Daten/pHGradienten/130403_Cy5_74mer_TRIS/130403_Cy5_74mer_TRIS/A_50mM_TRIS/50mA/TRIS_50mM_50mA_000284.tif", path "C:/Daten/pHGradienten/130403_Cy5_74mer_TRIS/130403_Cy5_74mer_TRIS/A_50mM_TRIS/50mA/TRIS_50mM_50mA_000285.tif", path "C:/Daten/pHGradienten/130403_Cy5_74mer_TRIS/130403_Cy5_74mer_TRIS/A_50mM_TRIS/50mA/TRIS_50mM_50mA_000286.tif", path "C:/Daten/pHGradienten/130403_Cy5_74mer_TRIS/130403_Cy5_74mer_TRIS/A_50mM_TRIS/50mA/TRIS_50mM_50mA_000287.tif", path "C:/Daten/pHGradienten/130403_Cy5_74mer_TRIS/130403_Cy5_74mer_TRIS/A_50mM_TRIS/50mA/TRIS_50mM_50mA_000288.tif", path "C:/Daten/pHGradienten/130403_Cy5_74mer_TRIS/130403_Cy5_74mer_TRIS/A_50mM_TRIS/50mA/TRIS_50mM_50mA_000289.tif", path "C:/Daten/pHGradienten/130403_Cy5_74mer_TRIS/130403_Cy5_74mer_TRIS/A_50mM_TRIS/50mA/TRIS_50mM_50mA_000290.tif", path "C:/Daten/pHGradienten/130403_Cy5_74mer_TRIS/130403_Cy5_74mer_TRIS/A_50mM_TRIS/50mA/TRIS_50mM_50mA_000291.tif", path "C:/Daten/pHGradienten/130403_Cy5_74mer_TRIS/130403_Cy5_74mer_TRIS/A_50mM_TRIS/50mA/TRIS_50mM_50mA_000292.tif", path "C:/Daten/pHGradienten/130403_Cy5_74mer_TRIS/130403_Cy5_74mer_TRIS/A_50mM_TRIS/50mA/TRIS_50mM_50mA_000293.tif", path "C:/Daten/pHGradienten/130403_Cy5_74mer_TRIS/130403_Cy5_74mer_TRIS/A_50mM_TRIS/50mA/TRIS_50mM_50mA_000294.tif", path "C:/Daten/pHGradienten/130403_Cy5_74mer_TRIS/130403_Cy5_74mer_TRIS/A_50mM_TRIS/50mA/TRIS_50mM_50mA_000295.tif", path "C:/Daten/pHGradienten/130403_Cy5_74mer_TRIS/130403_Cy5_74mer_TRIS/A_50mM_TRIS/50mA/TRIS_50mM_50mA_000296.tif", path "C:/Daten/pHGradienten/130403_Cy5_74mer_TRIS/130403_Cy5_74mer_TRIS/A_50mM_TRIS/50mA/TRIS_50mM_50mA_000297.tif", path "C:/Daten/pHGradienten/130403_Cy5_74mer_TRIS/130403_Cy5_74mer_TRIS/A_50mM_TRIS/50mA/TRIS_50mM_50mA_000298.tif", path "C:/Daten/pHGradienten/130403_Cy5_74mer_TRIS/130403_Cy5_74mer_TRIS/A_50mM_TRIS/50mA/TRIS_50mM_50mA_000299.tif", path "C:/Daten/pHGradienten/130403_Cy5_74mer_TRIS/130403_Cy5_74mer_TRIS/A_50mM_TRIS/50mA/TRIS_50mM_50mA_000300.tif", path "C:/Daten/pHGradienten/130403_Cy5_74mer_TRIS/130403_Cy5_74mer_TRIS/A_50mM_TRIS/50mA/TRIS_50mM_50mA_000301.tif", path "C:/Daten/pHGradienten/130403_Cy5_74mer_TRIS/130403_Cy5_74mer_TRIS/A_50mM_TRIS/50mA/TRIS_50mM_50mA_000302.tif", path "C:/Daten/pHGradienten/130403_Cy5_74mer_TRIS/130403_Cy5_74mer_TRIS/A_50mM_TRIS/50mA/TRIS_50mM_50mA_000303.tif", path "C:/Daten/pHGradienten/130403_Cy5_74mer_TRIS/130403_Cy5_74mer_TRIS/A_50mM_TRIS/50mA/TRIS_50mM_50mA_000304.tif", path "C:/Daten/pHGradienten/130403_Cy5_74mer_TRIS/130403_Cy5_74mer_TRIS/A_50mM_TRIS/50mA/TRIS_50mM_50mA_000305.tif", path "C:/Daten/pHGradienten/130403_Cy5_74mer_TRIS/130403_Cy5_74mer_TRIS/A_50mM_TRIS/50mA/TRIS_50mM_50mA_000306.tif", path "C:/Daten/pHGradienten/130403_Cy5_74mer_TRIS/130403_Cy5_74mer_TRIS/A_50mM_TRIS/50mA/TRIS_50mM_50mA_000307.tif", path "C:/Daten/pHGradienten/130403_Cy5_74mer_TRIS/130403_Cy5_74mer_TRIS/A_50mM_TRIS/50mA/TRIS_50mM_50mA_000308.tif", path "C:/Daten/pHGradienten/130403_Cy5_74mer_TRIS/130403_Cy5_74mer_TRIS/A_50mM_TRIS/50mA/TRIS_50mM_50mA_000309.tif", path "C:/Daten/pHGradienten/130403_Cy5_74mer_TRIS/130403_Cy5_74mer_TRIS/A_50mM_TRIS/50mA/TRIS_50mM_50mA_000310.tif", path "C:/Daten/pHGradienten/130403_Cy5_74mer_TRIS/130403_Cy5_74mer_TRIS/A_50mM_TRIS/50mA/TRIS_50mM_50mA_000311.tif", path "C:/Daten/pHGradienten/130403_Cy5_74mer_TRIS/130403_Cy5_74mer_TRIS/A_50mM_TRIS/50mA/TRIS_50mM_50mA_000312.tif", path "C:/Daten/pHGradienten/130403_Cy5_74mer_TRIS/130403_Cy5_74mer_TRIS/A_50mM_TRIS/50mA/TRIS_50mM_50mA_000313.tif", path "C:/Daten/pHGradienten/130403_Cy5_74mer_TRIS/130403_Cy5_74mer_TRIS/A_50mM_TRIS/50mA/TRIS_50mM_50mA_000314.tif", path "C:/Daten/pHGradienten/130403_Cy5_74mer_TRIS/130403_Cy5_74mer_TRIS/A_50mM_TRIS/50mA/TRIS_50mM_50mA_000315.tif", path "C:/Daten/pHGradienten/130403_Cy5_74mer_TRIS/130403_Cy5_74mer_TRIS/A_50mM_TRIS/50mA/TRIS_50mM_50mA_000316.tif", path "C:/Daten/pHGradienten/130403_Cy5_74mer_TRIS/130403_Cy5_74mer_TRIS/A_50mM_TRIS/50mA/TRIS_50mM_50mA_000317.tif", path "C:/Daten/pHGradienten/130403_Cy5_74mer_TRIS/130403_Cy5_74mer_TRIS/A_50mM_TRIS/50mA/TRIS_50mM_50mA_000318.tif", path "C:/Daten/pHGradienten/130403_Cy5_74mer_TRIS/130403_Cy5_74mer_TRIS/A_50mM_TRIS/50mA/TRIS_50mM_50mA_000319.tif", path "C:/Daten/pHGradienten/130403_Cy5_74mer_TRIS/130403_Cy5_74mer_TRIS/A_50mM_TRIS/50mA/TRIS_50mM_50mA_000320.tif", path "C:/Daten/pHGradienten/130403_Cy5_74mer_TRIS/130403_Cy5_74mer_TRIS/A_50mM_TRIS/50mA/TRIS_50mM_50mA_000321.tif", path "C:/Daten/pHGradienten/130403_Cy5_74mer_TRIS/130403_Cy5_74mer_TRIS/A_50mM_TRIS/50mA/TRIS_50mM_50mA_000322.tif", path "C:/Daten/pHGradienten/130403_Cy5_74mer_TRIS/130403_Cy5_74mer_TRIS/A_50mM_TRIS/50mA/TRIS_50mM_50mA_000323.tif", path "C:/Daten/pHGradienten/130403_Cy5_74mer_TRIS/130403_Cy5_74mer_TRIS/A_50mM_TRIS/50mA/TRIS_50mM_50mA_000324.tif", path "C:/Daten/pHGradienten/130403_Cy5_74mer_TRIS/130403_Cy5_74mer_TRIS/A_50mM_TRIS/50mA/TRIS_50mM_50mA_000325.tif", path "C:/Daten/pHGradienten/130403_Cy5_74mer_TRIS/130403_Cy5_74mer_TRIS/A_50mM_TRIS/50mA/TRIS_50mM_50mA_000326.tif", path "C:/Daten/pHGradienten/130403_Cy5_74mer_TRIS/130403_Cy5_74mer_TRIS/A_50mM_TRIS/50mA/TRIS_50mM_50mA_000327.tif", path "C:/Daten/pHGradienten/130403_Cy5_74mer_TRIS/130403_Cy5_74mer_TRIS/A_50mM_TRIS/50mA/TRIS_50mM_50mA_000328.tif", path "C:/Daten/pHGradienten/130403_Cy5_74mer_TRIS/130403_Cy5_74mer_TRIS/A_50mM_TRIS/50mA/TRIS_50mM_50mA_000329.tif", path "C:/Daten/pHGradienten/130403_Cy5_74mer_TRIS/130403_Cy5_74mer_TRIS/A_50mM_TRIS/50mA/TRIS_50mM_50mA_000330.tif", path "C:/Daten/pHGradienten/130403_Cy5_74mer_TRIS/130403_Cy5_74mer_TRIS/A_50mM_TRIS/50mA/TRIS_50mM_50mA_000331.tif", path "C:/Daten/pHGradienten/130403_Cy5_74mer_TRIS/130403_Cy5_74mer_TRIS/A_50mM_TRIS/50mA/TRIS_50mM_50mA_000332.tif", path "C:/Daten/pHGradienten/130403_Cy5_74mer_TRIS/130403_Cy5_74mer_TRIS/A_50mM_TRIS/50mA/TRIS_50mM_50mA_000333.tif", path "C:/Daten/pHGradienten/130403_Cy5_74mer_TRIS/130403_Cy5_74mer_TRIS/A_50mM_TRIS/50mA/TRIS_50mM_50mA_000334.tif", path "C:/Daten/pHGradienten/130403_Cy5_74mer_TRIS/130403_Cy5_74mer_TRIS/A_50mM_TRIS/50mA/TRIS_50mM_50mA_000335.tif", path "C:/Daten/pHGradienten/130403_Cy5_74mer_TRIS/130403_Cy5_74mer_TRIS/A_50mM_TRIS/50mA/TRIS_50mM_50mA_000336.tif", path "C:/Daten/pHGradienten/130403_Cy5_74mer_TRIS/130403_Cy5_74mer_TRIS/A_50mM_TRIS/50mA/TRIS_50mM_50mA_000337.tif", path "C:/Daten/pHGradienten/130403_Cy5_74mer_TRIS/130403_Cy5_74mer_TRIS/A_50mM_TRIS/50mA/TRIS_50mM_50mA_000338.tif", path "C:/Daten/pHGradienten/130403_Cy5_74mer_TRIS/130403_Cy5_74mer_TRIS/A_50mM_TRIS/50mA/TRIS_50mM_50mA_000339.tif", path "C:/Daten/pHGradienten/130403_Cy5_74mer_TRIS/130403_Cy5_74mer_TRIS/A_50mM_TRIS/50mA/TRIS_50mM_50mA_000340.tif", path "C:/Daten/pHGradienten/130403_Cy5_74mer_TRIS/130403_Cy5_74mer_TRIS/A_50mM_TRIS/50mA/TRIS_50mM_50mA_000341.tif", path "C:/Daten/pHGradienten/130403_Cy5_74mer_TRIS/130403_Cy5_74mer_TRIS/A_50mM_TRIS/50mA/TRIS_50mM_50mA_000342.tif", path "C:/Daten/pHGradienten/130403_Cy5_74mer_TRIS/130403_Cy5_74mer_TRIS/A_50mM_TRIS/50mA/TRIS_50mM_50mA_000343.tif", path "C:/Daten/pHGradienten/130403_Cy5_74mer_TRIS/130403_Cy5_74mer_TRIS/A_50mM_TRIS/50mA/TRIS_50mM_50mA_000344.tif", path "C:/Daten/pHGradienten/130403_Cy5_74mer_TRIS/130403_Cy5_74mer_TRIS/A_50mM_TRIS/50mA/TRIS_50mM_50mA_000345.tif", path "C:/Daten/pHGradienten/130403_Cy5_74mer_TRIS/130403_Cy5_74mer_TRIS/A_50mM_TRIS/50mA/TRIS_50mM_50mA_000346.tif", path "C:/Daten/pHGradienten/130403_Cy5_74mer_TRIS/130403_Cy5_74mer_TRIS/A_50mM_TRIS/50mA/TRIS_50mM_50mA_000347.tif", path "C:/Daten/pHGradienten/130403_Cy5_74mer_TRIS/130403_Cy5_74mer_TRIS/A_50mM_TRIS/50mA/TRIS_50mM_50mA_000348.tif", path "C:/Daten/pHGradienten/130403_Cy5_74mer_TRIS/130403_Cy5_74mer_TRIS/A_50mM_TRIS/50mA/TRIS_50mM_50mA_000349.tif", path "C:/Daten/pHGradienten/130403_Cy5_74mer_TRIS/130403_Cy5_74mer_TRIS/A_50mM_TRIS/50mA/TRIS_50mM_50mA_000350.tif", path "C:/Daten/pHGradienten/130403_Cy5_74mer_TRIS/130403_Cy5_74mer_TRIS/A_50mM_TRIS/50mA/TRIS_50mM_50mA_000351.tif", path "C:/Daten/pHGradienten/130403_Cy5_74mer_TRIS/130403_Cy5_74mer_TRIS/A_50mM_TRIS/50mA/TRIS_50mM_50mA_000352.tif", path "C:/Daten/pHGradienten/130403_Cy5_74mer_TRIS/130403_Cy5_74mer_TRIS/A_50mM_TRIS/50mA/TRIS_50mM_50mA_000353.tif", path "C:/Daten/pHGradienten/130403_Cy5_74mer_TRIS/130403_Cy5_74mer_TRIS/A_50mM_TRIS/50mA/TRIS_50mM_50mA_000354.tif", path "C:/Daten/pHGradienten/130403_Cy5_74mer_TRIS/130403_Cy5_74mer_TRIS/A_50mM_TRIS/50mA/TRIS_50mM_50mA_000355.tif", path "C:/Daten/pHGradienten/130403_Cy5_74mer_TRIS/130403_Cy5_74mer_TRIS/A_50mM_TRIS/50mA/TRIS_50mM_50mA_000356.tif", path "C:/Daten/pHGradienten/130403_Cy5_74mer_TRIS/130403_Cy5_74mer_TRIS/A_50mM_TRIS/50mA/TRIS_50mM_50mA_000357.tif", path "C:/Daten/pHGradienten/130403_Cy5_74mer_TRIS/130403_Cy5_74mer_TRIS/A_50mM_TRIS/50mA/TRIS_50mM_50mA_000358.tif", path "C:/Daten/pHGradienten/130403_Cy5_74mer_TRIS/130403_Cy5_74mer_TRIS/A_50mM_TRIS/50mA/TRIS_50mM_50mA_000359.tif", path "C:/Daten/pHGradienten/130403_Cy5_74mer_TRIS/130403_Cy5_74mer_TRIS/A_50mM_TRIS/50mA/TRIS_50mM_50mA_000360.tif", path "C:/Daten/pHGradienten/130403_Cy5_74mer_TRIS/130403_Cy5_74mer_TRIS/A_50mM_TRIS/50mA/TRIS_50mM_50mA_000361.tif", path "C:/Daten/pHGradienten/130403_Cy5_74mer_TRIS/130403_Cy5_74mer_TRIS/A_50mM_TRIS/50mA/TRIS_50mM_50mA_000362.tif", path "C:/Daten/pHGradienten/130403_Cy5_74mer_TRIS/130403_Cy5_74mer_TRIS/A_50mM_TRIS/50mA/TRIS_50mM_50mA_000363.tif", path "C:/Daten/pHGradienten/130403_Cy5_74mer_TRIS/130403_Cy5_74mer_TRIS/A_50mM_TRIS/50mA/TRIS_50mM_50mA_000364.tif", path "C:/Daten/pHGradienten/130403_Cy5_74mer_TRIS/130403_Cy5_74mer_TRIS/A_50mM_TRIS/50mA/TRIS_50mM_50mA_000365.tif", path "C:/Daten/pHGradienten/130403_Cy5_74mer_TRIS/130403_Cy5_74mer_TRIS/A_50mM_TRIS/50mA/TRIS_50mM_50mA_000366.tif", path "C:/Daten/pHGradienten/130403_Cy5_74mer_TRIS/130403_Cy5_74mer_TRIS/A_50mM_TRIS/50mA/TRIS_50mM_50mA_000367.tif", path "C:/Daten/pHGradienten/130403_Cy5_74mer_TRIS/130403_Cy5_74mer_TRIS/A_50mM_TRIS/50mA/TRIS_50mM_50mA_000368.tif", path "C:/Daten/pHGradienten/130403_Cy5_74mer_TRIS/130403_Cy5_74mer_TRIS/A_50mM_TRIS/50mA/TRIS_50mM_50mA_000369.tif", path "C:/Daten/pHGradienten/130403_Cy5_74mer_TRIS/130403_Cy5_74mer_TRIS/A_50mM_TRIS/50mA/TRIS_50mM_50mA_000370.tif", path "C:/Daten/pHGradienten/130403_Cy5_74mer_TRIS/130403_Cy5_74mer_TRIS/A_50mM_TRIS/50mA/TRIS_50mM_50mA_000371.tif", path "C:/Daten/pHGradienten/130403_Cy5_74mer_TRIS/130403_Cy5_74mer_TRIS/A_50mM_TRIS/50mA/TRIS_50mM_50mA_000372.tif", path "C:/Daten/pHGradienten/130403_Cy5_74mer_TRIS/130403_Cy5_74mer_TRIS/A_50mM_TRIS/50mA/TRIS_50mM_50mA_000373.tif", path "C:/Daten/pHGradienten/130403_Cy5_74mer_TRIS/130403_Cy5_74mer_TRIS/A_50mM_TRIS/50mA/TRIS_50mM_50mA_000374.tif", path "C:/Daten/pHGradienten/130403_Cy5_74mer_TRIS/130403_Cy5_74mer_TRIS/A_50mM_TRIS/50mA/TRIS_50mM_50mA_000375.tif", path "C:/Daten/pHGradienten/130403_Cy5_74mer_TRIS/130403_Cy5_74mer_TRIS/A_50mM_TRIS/50mA/TRIS_50mM_50mA_000376.tif", path "C:/Daten/pHGradienten/130403_Cy5_74mer_TRIS/130403_Cy5_74mer_TRIS/A_50mM_TRIS/50mA/TRIS_50mM_50mA_000377.tif", path "C:/Daten/pHGradienten/130403_Cy5_74mer_TRIS/130403_Cy5_74mer_TRIS/A_50mM_TRIS/50mA/TRIS_50mM_50mA_000378.tif", path "C:/Daten/pHGradienten/130403_Cy5_74mer_TRIS/130403_Cy5_74mer_TRIS/A_50mM_TRIS/50mA/TRIS_50mM_50mA_000379.tif", path "C:/Daten/pHGradienten/130403_Cy5_74mer_TRIS/130403_Cy5_74mer_TRIS/A_50mM_TRIS/50mA/TRIS_50mM_50mA_000380.tif", path "C:/Daten/pHGradienten/130403_Cy5_74mer_TRIS/130403_Cy5_74mer_TRIS/A_50mM_TRIS/50mA/TRIS_50mM_50mA_000381.tif", path "C:/Daten/pHGradienten/130403_Cy5_74mer_TRIS/130403_Cy5_74mer_TRIS/A_50mM_TRIS/50mA/TRIS_50mM_50mA_000382.tif", path "C:/Daten/pHGradienten/130403_Cy5_74mer_TRIS/130403_Cy5_74mer_TRIS/A_50mM_TRIS/50mA/TRIS_50mM_50mA_000383.tif", path "C:/Daten/pHGradienten/130403_Cy5_74mer_TRIS/130403_Cy5_74mer_TRIS/A_50mM_TRIS/50mA/TRIS_50mM_50mA_000384.tif", path "C:/Daten/pHGradienten/130403_Cy5_74mer_TRIS/130403_Cy5_74mer_TRIS/A_50mM_TRIS/50mA/TRIS_50mM_50mA_000385.tif", path "C:/Daten/pHGradienten/130403_Cy5_74mer_TRIS/130403_Cy5_74mer_TRIS/A_50mM_TRIS/50mA/TRIS_50mM_50mA_000386.tif", path "C:/Daten/pHGradienten/130403_Cy5_74mer_TRIS/130403_Cy5_74mer_TRIS/A_50mM_TRIS/50mA/TRIS_50mM_50mA_000387.tif", path "C:/Daten/pHGradienten/130403_Cy5_74mer_TRIS/130403_Cy5_74mer_TRIS/A_50mM_TRIS/50mA/TRIS_50mM_50mA_000388.tif", path "C:/Daten/pHGradienten/130403_Cy5_74mer_TRIS/130403_Cy5_74mer_TRIS/A_50mM_TRIS/50mA/TRIS_50mM_50mA_000389.tif", path "C:/Daten/pHGradienten/130403_Cy5_74mer_TRIS/130403_Cy5_74mer_TRIS/A_50mM_TRIS/50mA/TRIS_50mM_50mA_000390.tif", path "C:/Daten/pHGradienten/130403_Cy5_74mer_TRIS/130403_Cy5_74mer_TRIS/A_50mM_TRIS/50mA/TRIS_50mM_50mA_000391.tif", path "C:/Daten/pHGradienten/130403_Cy5_74mer_TRIS/130403_Cy5_74mer_TRIS/A_50mM_TRIS/50mA/TRIS_50mM_50mA_000392.tif", path "C:/Daten/pHGradienten/130403_Cy5_74mer_TRIS/130403_Cy5_74mer_TRIS/A_50mM_TRIS/50mA/TRIS_50mM_50mA_000393.tif", path "C:/Daten/pHGradienten/130403_Cy5_74mer_TRIS/130403_Cy5_74mer_TRIS/A_50mM_TRIS/50mA/TRIS_50mM_50mA_000394.tif", path "C:/Daten/pHGradienten/130403_Cy5_74mer_TRIS/130403_Cy5_74mer_TRIS/A_50mM_TRIS/50mA/TRIS_50mM_50mA_000395.tif", path "C:/Daten/pHGradienten/130403_Cy5_74mer_TRIS/130403_Cy5_74mer_TRIS/A_50mM_TRIS/50mA/TRIS_50mM_50mA_000396.tif", path "C:/Daten/pHGradienten/130403_Cy5_74mer_TRIS/130403_Cy5_74mer_TRIS/A_50mM_TRIS/50mA/TRIS_50mM_50mA_000397.tif", path "C:/Daten/pHGradienten/130403_Cy5_74mer_TRIS/130403_Cy5_74mer_TRIS/A_50mM_TRIS/50mA/TRIS_50mM_50mA_000398.tif", path "C:/Daten/pHGradienten/130403_Cy5_74mer_TRIS/130403_Cy5_74mer_TRIS/A_50mM_TRIS/50mA/TRIS_50mM_50mA_000399.tif"], 3 "Center Position [Pixel]":cluster{"Cursor X":dbl, "Cursor Y":dbl}={"Cursor X"=2.5, "Cursor Y"=2.5}, 5 "Background Path in Folder":path[](array[path])=[path "C:/Daten/pHGradienten/130403_Cy5_74mer_TRIS/130403_Cy5_74mer_TRIS/A_50mM_TRIS/50mA/TRIS_50mM_50mA_000001.tif", path "C:/Daten/pHGradienten/130403_Cy5_74mer_TRIS/130403_Cy5_74mer_TRIS/A_50mM_TRIS/50mA/TRIS_50mM_50mA_000002.tif", path "C:/Daten/pHGradienten/130403_Cy5_74mer_TRIS/130403_Cy5_74mer_TRIS/A_50mM_TRIS/50mA/TRIS_50mM_50mA_000003.tif", path "C:/Daten/pHGradienten/130403_Cy5_74mer_TRIS/130403_Cy5_74mer_TRIS/A_50mM_TRIS/50mA/TRIS_50mM_50mA_000004.tif", path "C:/Daten/pHGradienten/130403_Cy5_74mer_TRIS/130403_Cy5_74mer_TRIS/A_50mM_TRIS/50mA/TRIS_50mM_50mA_000005.tif", path "C:/Daten/pHGradienten/130403_Cy5_74mer_TRIS/130403_Cy5_74mer_TRIS/A_50mM_TRIS/50mA/TRIS_50mM_50mA_000006.tif", path "C:/Daten/pHGradienten/130403_Cy5_74mer_TRIS/130403_Cy5_74mer_TRIS/A_50mM_TRIS/50mA/TRIS_50mM_50mA_000007.tif", path "C:/Daten/pHGradienten/130403_Cy5_74mer_TRIS/130403_Cy5_74mer_TRIS/A_50mM_TRIS/50mA/TRIS_50mM_50mA_000008.tif", path "C:/Daten/pHGradienten/130403_Cy5_74mer_TRIS/130403_Cy5_74mer_TRIS/A_50mM_TRIS/50mA/TRIS_50mM_50mA_000009.tif", path "C:/Daten/pHGradienten/130403_Cy5_74mer_TRIS/130403_Cy5_74mer_TRIS/A_50mM_TRIS/50mA/TRIS_50mM_50mA_000010.tif", path "C:/Daten/pHGradienten/130403_Cy5_74mer_TRIS/130403_Cy5_74mer_TRIS/A_50mM_TRIS/50mA/TRIS_50mM_50mA_000011.tif", path "C:/Daten/pHGradienten/130403_Cy5_74mer_TRIS/130403_Cy5_74mer_TRIS/A_50mM_TRIS/50mA/TRIS_50mM_50mA_000012.tif", path "C:/Daten/pHGradienten/130403_Cy5_74mer_TRIS/130403_Cy5_74mer_TRIS/A_50mM_TRIS/50mA/TRIS_50mM_50mA_000013.tif", path "C:/Daten/pHGradienten/130403_Cy5_74mer_TRIS/130403_Cy5_74mer_TRIS/A_50mM_TRIS/50mA/TRIS_50mM_50mA_000014.tif", path "C:/Daten/pHGradienten/130403_Cy5_74mer_TRIS/130403_Cy5_74mer_TRIS/A_50mM_TRIS/50mA/TRIS_50mM_50mA_000015.tif", path "C:/Daten/pHGradienten/130403_Cy5_74mer_TRIS/130403_Cy5_74mer_TRIS/A_50mM_TRIS/50mA/TRIS_50mM_50mA_000016.tif", path "C:/Daten/pHGradienten/130403_Cy5_74mer_TRIS/130403_Cy5_74mer_TRIS/A_50mM_TRIS/50mA/TRIS_50mM_50mA_000017.tif", path "C:/Daten/pHGradienten/130403_Cy5_74mer_TRIS/130403_Cy5_74mer_TRIS/A_50mM_TRIS/50mA/TRIS_50mM_50mA_000018.tif", path "C:/Daten/pHGradienten/130403_Cy5_74mer_TRIS/130403_Cy5_74mer_TRIS/A_50mM_TRIS/50mA/TRIS_50mM_50mA_000019.tif", path "C:/Daten/pHGradienten/130403_Cy5_74mer_TRIS/130403_Cy5_74mer_TRIS/A_50mM_TRIS/50mA/TRIS_50mM_50mA_000020.tif", path "C:/Daten/pHGradienten/130403_Cy5_74mer_TRIS/130403_Cy5_74mer_TRIS/A_50mM_TRIS/50mA/TRIS_50mM_50mA_000021.tif", path "C:/Daten/pHGradienten/130403_Cy5_74mer_TRIS/130403_Cy5_74mer_TRIS/A_50mM_TRIS/50mA/TRIS_50mM_50mA_000022.tif", path "C:/Daten/pHGradienten/130403_Cy5_74mer_TRIS/130403_Cy5_74mer_TRIS/A_50mM_TRIS/50mA/TRIS_50mM_50mA_000023.tif", path "C:/Daten/pHGradienten/130403_Cy5_74mer_TRIS/130403_Cy5_74mer_TRIS/A_50mM_TRIS/50mA/TRIS_50mM_50mA_000024.tif", path "C:/Daten/pHGradienten/130403_Cy5_74mer_TRIS/130403_Cy5_74mer_TRIS/A_50mM_TRIS/50mA/TRIS_50mM_50mA_000025.tif", path "C:/Daten/pHGradienten/130403_Cy5_74mer_TRIS/130403_Cy5_74mer_TRIS/A_50mM_TRIS/50mA/TRIS_50mM_50mA_000026.tif", path "C:/Daten/pHGradienten/130403_Cy5_74mer_TRIS/130403_Cy5_74mer_TRIS/A_50mM_TRIS/50mA/TRIS_50mM_50mA_000027.tif", path "C:/Daten/pHGradienten/130403_Cy5_74mer_TRIS/130403_Cy5_74mer_TRIS/A_50mM_TRIS/50mA/TRIS_50mM_50mA_000028.tif", path "C:/Daten/pHGradienten/130403_Cy5_74mer_TRIS/130403_Cy5_74mer_TRIS/A_50mM_TRIS/50mA/TRIS_50mM_50mA_000029.tif", path "C:/Daten/pHGradienten/130403_Cy5_74mer_TRIS/130403_Cy5_74mer_TRIS/A_50mM_TRIS/50mA/TRIS_50mM_50mA_000030.tif", path "C:/Daten/pHGradienten/130403_Cy5_74mer_TRIS/130403_Cy5_74mer_TRIS/A_50mM_TRIS/50mA/TRIS_50mM_50mA_000031.tif", path "C:/Daten/pHGradienten/130403_Cy5_74mer_TRIS/130403_Cy5_74mer_TRIS/A_50mM_TRIS/50mA/TRIS_50mM_50mA_000032.tif", path "C:/Daten/pHGradienten/130403_Cy5_74mer_TRIS/130403_Cy5_74mer_TRIS/A_50mM_TRIS/50mA/TRIS_50mM_50mA_000033.tif", path "C:/Daten/pHGradienten/130403_Cy5_74mer_TRIS/130403_Cy5_74mer_TRIS/A_50mM_TRIS/50mA/TRIS_50mM_50mA_000034.tif", path "C:/Daten/pHGradienten/130403_Cy5_74mer_TRIS/130403_Cy5_74mer_TRIS/A_50mM_TRIS/50mA/TRIS_50mM_50mA_000035.tif", path "C:/Daten/pHGradienten/130403_Cy5_74mer_TRIS/130403_Cy5_74mer_TRIS/A_50mM_TRIS/50mA/TRIS_50mM_50mA_000036.tif", path "C:/Daten/pHGradienten/130403_Cy5_74mer_TRIS/130403_Cy5_74mer_TRIS/A_50mM_TRIS/50mA/TRIS_50mM_50mA_000037.tif", path "C:/Daten/pHGradienten/130403_Cy5_74mer_TRIS/130403_Cy5_74mer_TRIS/A_50mM_TRIS/50mA/TRIS_50mM_50mA_000038.tif", path "C:/Daten/pHGradienten/130403_Cy5_74mer_TRIS/130403_Cy5_74mer_TRIS/A_50mM_TRIS/50mA/TRIS_50mM_50mA_000039.tif", path "C:/Daten/pHGradienten/130403_Cy5_74mer_TRIS/130403_Cy5_74mer_TRIS/A_50mM_TRIS/50mA/TRIS_50mM_50mA_000040.tif", path "C:/Daten/pHGradienten/130403_Cy5_74mer_TRIS/130403_Cy5_74mer_TRIS/A_50mM_TRIS/50mA/TRIS_50mM_50mA_000041.tif", path "C:/Daten/pHGradienten/130403_Cy5_74mer_TRIS/130403_Cy5_74mer_TRIS/A_50mM_TRIS/50mA/TRIS_50mM_50mA_000042.tif", path "C:/Daten/pHGradienten/130403_Cy5_74mer_TRIS/130403_Cy5_74mer_TRIS/A_50mM_TRIS/50mA/TRIS_50mM_50mA_000043.tif", path "C:/Daten/pHGradienten/130403_Cy5_74mer_TRIS/130403_Cy5_74mer_TRIS/A_50mM_TRIS/50mA/TRIS_50mM_50mA_000044.tif", path "C:/Daten/pHGradienten/130403_Cy5_74mer_TRIS/130403_Cy5_74mer_TRIS/A_50mM_TRIS/50mA/TRIS_50mM_50mA_000045.tif", path "C:/Daten/pHGradienten/130403_Cy5_74mer_TRIS/130403_Cy5_74mer_TRIS/A_50mM_TRIS/50mA/TRIS_50mM_50mA_000046.tif", path "C:/Daten/pHGradienten/130403_Cy5_74mer_TRIS/130403_Cy5_74mer_TRIS/A_50mM_TRIS/50mA/TRIS_50mM_50mA_000047.tif", path "C:/Daten/pHGradienten/130403_Cy5_74mer_TRIS/130403_Cy5_74mer_TRIS/A_50mM_TRIS/50mA/TRIS_50mM_50mA_000048.tif", path "C:/Daten/pHGradienten/130403_Cy5_74mer_TRIS/130403_Cy5_74mer_TRIS/A_50mM_TRIS/50mA/TRIS_50mM_50mA_000049.tif", path "C:/Daten/pHGradienten/130403_Cy5_74mer_TRIS/130403_Cy5_74mer_TRIS/A_50mM_TRIS/50mA/TRIS_50mM_50mA_000050.tif", path "C:/Daten/pHGradienten/130403_Cy5_74mer_TRIS/130403_Cy5_74mer_TRIS/A_50mM_TRIS/50mA/TRIS_50mM_50mA_000051.tif", path "C:/Daten/pHGradienten/130403_Cy5_74mer_TRIS/130403_Cy5_74mer_TRIS/A_50mM_TRIS/50mA/TRIS_50mM_50mA_000052.tif", path "C:/Daten/pHGradienten/130403_Cy5_74mer_TRIS/130403_Cy5_74mer_TRIS/A_50mM_TRIS/50mA/TRIS_50mM_50mA_000053.tif", path "C:/Daten/pHGradienten/130403_Cy5_74mer_TRIS/130403_Cy5_74mer_TRIS/A_50mM_TRIS/50mA/TRIS_50mM_50mA_000054.tif", path "C:/Daten/pHGradienten/130403_Cy5_74mer_TRIS/130403_Cy5_74mer_TRIS/A_50mM_TRIS/50mA/TRIS_50mM_50mA_000055.tif", path "C:/Daten/pHGradienten/130403_Cy5_74mer_TRIS/130403_Cy5_74mer_TRIS/A_50mM_TRIS/50mA/TRIS_50mM_50mA_000056.tif", path "C:/Daten/pHGradienten/130403_Cy5_74mer_TRIS/130403_Cy5_74mer_TRIS/A_50mM_TRIS/50mA/TRIS_50mM_50mA_000057.tif", path "C:/Daten/pHGradienten/130403_Cy5_74mer_TRIS/130403_Cy5_74mer_TRIS/A_50mM_TRIS/50mA/TRIS_50mM_50mA_000058.tif", path "C:/Daten/pHGradienten/130403_Cy5_74mer_TRIS/130403_Cy5_74mer_TRIS/A_50mM_TRIS/50mA/TRIS_50mM_50mA_000059.tif", path "C:/Daten/pHGradienten/130403_Cy5_74mer_TRIS/130403_Cy5_74mer_TRIS/A_50mM_TRIS/50mA/TRIS_50mM_50mA_000060.tif", path "C:/Daten/pHGradienten/130403_Cy5_74mer_TRIS/130403_Cy5_74mer_TRIS/A_50mM_TRIS/50mA/TRIS_50mM_50mA_000061.tif", path "C:/Daten/pHGradienten/130403_Cy5_74mer_TRIS/130403_Cy5_74mer_TRIS/A_50mM_TRIS/50mA/TRIS_50mM_50mA_000062.tif", path "C:/Daten/pHGradienten/130403_Cy5_74mer_TRIS/130403_Cy5_74mer_TRIS/A_50mM_TRIS/50mA/TRIS_50mM_50mA_000063.tif", path "C:/Daten/pHGradienten/130403_Cy5_74mer_TRIS/130403_Cy5_74mer_TRIS/A_50mM_TRIS/50mA/TRIS_50mM_50mA_000064.tif", path "C:/Daten/pHGradienten/130403_Cy5_74mer_TRIS/130403_Cy5_74mer_TRIS/A_50mM_TRIS/50mA/TRIS_50mM_50mA_000065.tif", path "C:/Daten/pHGradienten/130403_Cy5_74mer_TRIS/130403_Cy5_74mer_TRIS/A_50mM_TRIS/50mA/TRIS_50mM_50mA_000066.tif", path "C:/Daten/pHGradienten/130403_Cy5_74mer_TRIS/130403_Cy5_74mer_TRIS/A_50mM_TRIS/50mA/TRIS_50mM_50mA_000067.tif", path "C:/Daten/pHGradienten/130403_Cy5_74mer_TRIS/130403_Cy5_74mer_TRIS/A_50mM_TRIS/50mA/TRIS_50mM_50mA_000068.tif", path "C:/Daten/pHGradienten/130403_Cy5_74mer_TRIS/130403_Cy5_74mer_TRIS/A_50mM_TRIS/50mA/TRIS_50mM_50mA_000069.tif", path "C:/Daten/pHGradienten/130403_Cy5_74mer_TRIS/130403_Cy5_74mer_TRIS/A_50mM_TRIS/50mA/TRIS_50mM_50mA_000070.tif", path "C:/Daten/pHGradienten/130403_Cy5_74mer_TRIS/130403_Cy5_74mer_TRIS/A_50mM_TRIS/50mA/TRIS_50mM_50mA_000071.tif", path "C:/Daten/pHGradienten/130403_Cy5_74mer_TRIS/130403_Cy5_74mer_TRIS/A_50mM_TRIS/50mA/TRIS_50mM_50mA_000072.tif", path "C:/Daten/pHGradienten/130403_Cy5_74mer_TRIS/130403_Cy5_74mer_TRIS/A_50mM_TRIS/50mA/TRIS_50mM_50mA_000073.tif", path "C:/Daten/pHGradienten/130403_Cy5_74mer_TRIS/130403_Cy5_74mer_TRIS/A_50mM_TRIS/50mA/TRIS_50mM_50mA_000074.tif", path "C:/Daten/pHGradienten/130403_Cy5_74mer_TRIS/130403_Cy5_74mer_TRIS/A_50mM_TRIS/50mA/TRIS_50mM_50mA_000075.tif", path "C:/Daten/pHGradienten/130403_Cy5_74mer_TRIS/130403_Cy5_74mer_TRIS/A_50mM_TRIS/50mA/TRIS_50mM_50mA_000076.tif", path "C:/Daten/pHGradienten/130403_Cy5_74mer_TRIS/130403_Cy5_74mer_TRIS/A_50mM_TRIS/50mA/TRIS_50mM_50mA_000077.tif", path "C:/Daten/pHGradienten/130403_Cy5_74mer_TRIS/130403_Cy5_74mer_TRIS/A_50mM_TRIS/50mA/TRIS_50mM_50mA_000078.tif", path "C:/Daten/pHGradienten/130403_Cy5_74mer_TRIS/130403_Cy5_74mer_TRIS/A_50mM_TRIS/50mA/TRIS_50mM_50mA_000079.tif", path "C:/Daten/pHGradienten/130403_Cy5_74mer_TRIS/130403_Cy5_74mer_TRIS/A_50mM_TRIS/50mA/TRIS_50mM_50mA_000080.tif", path "C:/Daten/pHGradienten/130403_Cy5_74mer_TRIS/130403_Cy5_74mer_TRIS/A_50mM_TRIS/50mA/TRIS_50mM_50mA_000081.tif", path "C:/Daten/pHGradienten/130403_Cy5_74mer_TRIS/130403_Cy5_74mer_TRIS/A_50mM_TRIS/50mA/TRIS_50mM_50mA_000082.tif", path "C:/Daten/pHGradienten/130403_Cy5_74mer_TRIS/130403_Cy5_74mer_TRIS/A_50mM_TRIS/50mA/TRIS_50mM_50mA_000083.tif", path "C:/Daten/pHGradienten/130403_Cy5_74mer_TRIS/130403_Cy5_74mer_TRIS/A_50mM_TRIS/50mA/TRIS_50mM_50mA_000084.tif", path "C:/Daten/pHGradienten/130403_Cy5_74mer_TRIS/130403_Cy5_74mer_TRIS/A_50mM_TRIS/50mA/TRIS_50mM_50mA_000085.tif", path "C:/Daten/pHGradienten/130403_Cy5_74mer_TRIS/130403_Cy5_74mer_TRIS/A_50mM_TRIS/50mA/TRIS_50mM_50mA_000086.tif", path "C:/Daten/pHGradienten/130403_Cy5_74mer_TRIS/130403_Cy5_74mer_TRIS/A_50mM_TRIS/50mA/TRIS_50mM_50mA_000087.tif", path "C:/Daten/pHGradienten/130403_Cy5_74mer_TRIS/130403_Cy5_74mer_TRIS/A_50mM_TRIS/50mA/TRIS_50mM_50mA_000088.tif", path "C:/Daten/pHGradienten/130403_Cy5_74mer_TRIS/130403_Cy5_74mer_TRIS/A_50mM_TRIS/50mA/TRIS_50mM_50mA_000089.tif", path "C:/Daten/pHGradienten/130403_Cy5_74mer_TRIS/130403_Cy5_74mer_TRIS/A_50mM_TRIS/50mA/TRIS_50mM_50mA_000090.tif", path "C:/Daten/pHGradienten/130403_Cy5_74mer_TRIS/130403_Cy5_74mer_TRIS/A_50mM_TRIS/50mA/TRIS_50mM_50mA_000091.tif", path "C:/Daten/pHGradienten/130403_Cy5_74mer_TRIS/130403_Cy5_74mer_TRIS/A_50mM_TRIS/50mA/TRIS_50mM_50mA_000092.tif", path "C:/Daten/pHGradienten/130403_Cy5_74mer_TRIS/130403_Cy5_74mer_TRIS/A_50mM_TRIS/50mA/TRIS_50mM_50mA_000093.tif", path "C:/Daten/pHGradienten/130403_Cy5_74mer_TRIS/130403_Cy5_74mer_TRIS/A_50mM_TRIS/50mA/TRIS_50mM_50mA_000094.tif", path "C:/Daten/pHGradienten/130403_Cy5_74mer_TRIS/130403_Cy5_74mer_TRIS/A_50mM_TRIS/50mA/TRIS_50mM_50mA_000095.tif", path "C:/Daten/pHGradienten/130403_Cy5_74mer_TRIS/130403_Cy5_74mer_TRIS/A_50mM_TRIS/50mA/TRIS_50mM_50mA_000096.tif", path "C:/Daten/pHGradienten/130403_Cy5_74mer_TRIS/130403_Cy5_74mer_TRIS/A_50mM_TRIS/50mA/TRIS_50mM_50mA_000097.tif", path "C:/Daten/pHGradienten/130403_Cy5_74mer_TRIS/130403_Cy5_74mer_TRIS/A_50mM_TRIS/50mA/TRIS_50mM_50mA_000098.tif", path "C:/Daten/pHGradienten/130403_Cy5_74mer_TRIS/130403_Cy5_74mer_TRIS/A_50mM_TRIS/50mA/TRIS_50mM_50mA_000099.tif", path "C:/Daten/pHGradienten/130403_Cy5_74mer_TRIS/130403_Cy5_74mer_TRIS/A_50mM_TRIS/50mA/TRIS_50mM_50mA_000100.tif", path "C:/Daten/pHGradienten/130403_Cy5_74mer_TRIS/130403_Cy5_74mer_TRIS/A_50mM_TRIS/50mA/TRIS_50mM_50mA_000101.tif", path "C:/Daten/pHGradienten/130403_Cy5_74mer_TRIS/130403_Cy5_74mer_TRIS/A_50mM_TRIS/50mA/TRIS_50mM_50mA_000102.tif", path "C:/Daten/pHGradienten/130403_Cy5_74mer_TRIS/130403_Cy5_74mer_TRIS/A_50mM_TRIS/50mA/TRIS_50mM_50mA_000103.tif", path "C:/Daten/pHGradienten/130403_Cy5_74mer_TRIS/130403_Cy5_74mer_TRIS/A_50mM_TRIS/50mA/TRIS_50mM_50mA_000104.tif", path "C:/Daten/pHGradienten/130403_Cy5_74mer_TRIS/130403_Cy5_74mer_TRIS/A_50mM_TRIS/50mA/TRIS_50mM_50mA_000105.tif", path "C:/Daten/pHGradienten/130403_Cy5_74mer_TRIS/130403_Cy5_74mer_TRIS/A_50mM_TRIS/50mA/TRIS_50mM_50mA_000106.tif", path "C:/Daten/pHGradienten/130403_Cy5_74mer_TRIS/130403_Cy5_74mer_TRIS/A_50mM_TRIS/50mA/TRIS_50mM_50mA_000107.tif", path "C:/Daten/pHGradienten/130403_Cy5_74mer_TRIS/130403_Cy5_74mer_TRIS/A_50mM_TRIS/50mA/TRIS_50mM_50mA_000108.tif", path "C:/Daten/pHGradienten/130403_Cy5_74mer_TRIS/130403_Cy5_74mer_TRIS/A_50mM_TRIS/50mA/TRIS_50mM_50mA_000109.tif", path "C:/Daten/pHGradienten/130403_Cy5_74mer_TRIS/130403_Cy5_74mer_TRIS/A_50mM_TRIS/50mA/TRIS_50mM_50mA_000110.tif", path "C:/Daten/pHGradienten/130403_Cy5_74mer_TRIS/130403_Cy5_74mer_TRIS/A_50mM_TRIS/50mA/TRIS_50mM_50mA_000111.tif", path "C:/Daten/pHGradienten/130403_Cy5_74mer_TRIS/130403_Cy5_74mer_TRIS/A_50mM_TRIS/50mA/TRIS_50mM_50mA_000112.tif", path "C:/Daten/pHGradienten/130403_Cy5_74mer_TRIS/130403_Cy5_74mer_TRIS/A_50mM_TRIS/50mA/TRIS_50mM_50mA_000113.tif", path "C:/Daten/pHGradienten/130403_Cy5_74mer_TRIS/130403_Cy5_74mer_TRIS/A_50mM_TRIS/50mA/TRIS_50mM_50mA_000114.tif", path "C:/Daten/pHGradienten/130403_Cy5_74mer_TRIS/130403_Cy5_74mer_TRIS/A_50mM_TRIS/50mA/TRIS_50mM_50mA_000115.tif", path "C:/Daten/pHGradienten/130403_Cy5_74mer_TRIS/130403_Cy5_74mer_TRIS/A_50mM_TRIS/50mA/TRIS_50mM_50mA_000116.tif", path "C:/Daten/pHGradienten/130403_Cy5_74mer_TRIS/130403_Cy5_74mer_TRIS/A_50mM_TRIS/50mA/TRIS_50mM_50mA_000117.tif", path "C:/Daten/pHGradienten/130403_Cy5_74mer_TRIS/130403_Cy5_74mer_TRIS/A_50mM_TRIS/50mA/TRIS_50mM_50mA_000118.tif", path "C:/Daten/pHGradienten/130403_Cy5_74mer_TRIS/130403_Cy5_74mer_TRIS/A_50mM_TRIS/50mA/TRIS_50mM_50mA_000119.tif", path "C:/Daten/pHGradienten/130403_Cy5_74mer_TRIS/130403_Cy5_74mer_TRIS/A_50mM_TRIS/50mA/TRIS_50mM_50mA_000120.tif", path "C:/Daten/pHGradienten/130403_Cy5_74mer_TRIS/130403_Cy5_74mer_TRIS/A_50mM_TRIS/50mA/TRIS_50mM_50mA_000121.tif", path "C:/Daten/pHGradienten/130403_Cy5_74mer_TRIS/130403_Cy5_74mer_TRIS/A_50mM_TRIS/50mA/TRIS_50mM_50mA_000122.tif", path "C:/Daten/pHGradienten/130403_Cy5_74mer_TRIS/130403_Cy5_74mer_TRIS/A_50mM_TRIS/50mA/TRIS_50mM_50mA_000123.tif", path "C:/Daten/pHGradienten/130403_Cy5_74mer_TRIS/130403_Cy5_74mer_TRIS/A_50mM_TRIS/50mA/TRIS_50mM_50mA_000124.tif", path "C:/Daten/pHGradienten/130403_Cy5_74mer_TRIS/130403_Cy5_74mer_TRIS/A_50mM_TRIS/50mA/TRIS_50mM_50mA_000125.tif", path "C:/Daten/pHGradienten/130403_Cy5_74mer_TRIS/130403_Cy5_74mer_TRIS/A_50mM_TRIS/50mA/TRIS_50mM_50mA_000126.tif", path "C:/Daten/pHGradienten/130403_Cy5_74mer_TRIS/130403_Cy5_74mer_TRIS/A_50mM_TRIS/50mA/TRIS_50mM_50mA_000127.tif", path "C:/Daten/pHGradienten/130403_Cy5_74mer_TRIS/130403_Cy5_74mer_TRIS/A_50mM_TRIS/50mA/TRIS_50mM_50mA_000128.tif", path "C:/Daten/pHGradienten/130403_Cy5_74mer_TRIS/130403_Cy5_74mer_TRIS/A_50mM_TRIS/50mA/TRIS_50mM_50mA_000129.tif", path "C:/Daten/pHGradienten/130403_Cy5_74mer_TRIS/130403_Cy5_74mer_TRIS/A_50mM_TRIS/50mA/TRIS_50mM_50mA_000130.tif", path "C:/Daten/pHGradienten/130403_Cy5_74mer_TRIS/130403_Cy5_74mer_TRIS/A_50mM_TRIS/50mA/TRIS_50mM_50mA_000131.tif", path "C:/Daten/pHGradienten/130403_Cy5_74mer_TRIS/130403_Cy5_74mer_TRIS/A_50mM_TRIS/50mA/TRIS_50mM_50mA_000132.tif", path "C:/Daten/pHGradienten/130403_Cy5_74mer_TRIS/130403_Cy5_74mer_TRIS/A_50mM_TRIS/50mA/TRIS_50mM_50mA_000133.tif", path "C:/Daten/pHGradienten/130403_Cy5_74mer_TRIS/130403_Cy5_74mer_TRIS/A_50mM_TRIS/50mA/TRIS_50mM_50mA_000134.tif", path "C:/Daten/pHGradienten/130403_Cy5_74mer_TRIS/130403_Cy5_74mer_TRIS/A_50mM_TRIS/50mA/TRIS_50mM_50mA_000135.tif", path "C:/Daten/pHGradienten/130403_Cy5_74mer_TRIS/130403_Cy5_74mer_TRIS/A_50mM_TRIS/50mA/TRIS_50mM_50mA_000136.tif", path "C:/Daten/pHGradienten/130403_Cy5_74mer_TRIS/130403_Cy5_74mer_TRIS/A_50mM_TRIS/50mA/TRIS_50mM_50mA_000137.tif", path "C:/Daten/pHGradienten/130403_Cy5_74mer_TRIS/130403_Cy5_74mer_TRIS/A_50mM_TRIS/50mA/TRIS_50mM_50mA_000138.tif", path "C:/Daten/pHGradienten/130403_Cy5_74mer_TRIS/130403_Cy5_74mer_TRIS/A_50mM_TRIS/50mA/TRIS_50mM_50mA_000139.tif", path "C:/Daten/pHGradienten/130403_Cy5_74mer_TRIS/130403_Cy5_74mer_TRIS/A_50mM_TRIS/50mA/TRIS_50mM_50mA_000140.tif", path "C:/Daten/pHGradienten/130403_Cy5_74mer_TRIS/130403_Cy5_74mer_TRIS/A_50mM_TRIS/50mA/TRIS_50mM_50mA_000141.tif", path "C:/Daten/pHGradienten/130403_Cy5_74mer_TRIS/130403_Cy5_74mer_TRIS/A_50mM_TRIS/50mA/TRIS_50mM_50mA_000142.tif", path "C:/Daten/pHGradienten/130403_Cy5_74mer_TRIS/130403_Cy5_74mer_TRIS/A_50mM_TRIS/50mA/TRIS_50mM_50mA_000143.tif", path "C:/Daten/pHGradienten/130403_Cy5_74mer_TRIS/130403_Cy5_74mer_TRIS/A_50mM_TRIS/50mA/TRIS_50mM_50mA_000144.tif", path "C:/Daten/pHGradienten/130403_Cy5_74mer_TRIS/130403_Cy5_74mer_TRIS/A_50mM_TRIS/50mA/TRIS_50mM_50mA_000145.tif", path "C:/Daten/pHGradienten/130403_Cy5_74mer_TRIS/130403_Cy5_74mer_TRIS/A_50mM_TRIS/50mA/TRIS_50mM_50mA_000146.tif", path "C:/Daten/pHGradienten/130403_Cy5_74mer_TRIS/130403_Cy5_74mer_TRIS/A_50mM_TRIS/50mA/TRIS_50mM_50mA_000147.tif", path "C:/Daten/pHGradienten/130403_Cy5_74mer_TRIS/130403_Cy5_74mer_TRIS/A_50mM_TRIS/50mA/TRIS_50mM_50mA_000148.tif", path "C:/Daten/pHGradienten/130403_Cy5_74mer_TRIS/130403_Cy5_74mer_TRIS/A_50mM_TRIS/50mA/TRIS_50mM_50mA_000149.tif", path "C:/Daten/pHGradienten/130403_Cy5_74mer_TRIS/130403_Cy5_74mer_TRIS/A_50mM_TRIS/50mA/TRIS_50mM_50mA_000150.tif", path "C:/Daten/pHGradienten/130403_Cy5_74mer_TRIS/130403_Cy5_74mer_TRIS/A_50mM_TRIS/50mA/TRIS_50mM_50mA_000151.tif", path "C:/Daten/pHGradienten/130403_Cy5_74mer_TRIS/130403_Cy5_74mer_TRIS/A_50mM_TRIS/50mA/TRIS_50mM_50mA_000152.tif", path "C:/Daten/pHGradienten/130403_Cy5_74mer_TRIS/130403_Cy5_74mer_TRIS/A_50mM_TRIS/50mA/TRIS_50mM_50mA_000153.tif", path "C:/Daten/pHGradienten/130403_Cy5_74mer_TRIS/130403_Cy5_74mer_TRIS/A_50mM_TRIS/50mA/TRIS_50mM_50mA_000154.tif", path "C:/Daten/pHGradienten/130403_Cy5_74mer_TRIS/130403_Cy5_74mer_TRIS/A_50mM_TRIS/50mA/TRIS_50mM_50mA_000155.tif", path "C:/Daten/pHGradienten/130403_Cy5_74mer_TRIS/130403_Cy5_74mer_TRIS/A_50mM_TRIS/50mA/TRIS_50mM_50mA_000156.tif", path "C:/Daten/pHGradienten/130403_Cy5_74mer_TRIS/130403_Cy5_74mer_TRIS/A_50mM_TRIS/50mA/TRIS_50mM_50mA_000157.tif", path "C:/Daten/pHGradienten/130403_Cy5_74mer_TRIS/130403_Cy5_74mer_TRIS/A_50mM_TRIS/50mA/TRIS_50mM_50mA_000158.tif", path "C:/Daten/pHGradienten/130403_Cy5_74mer_TRIS/130403_Cy5_74mer_TRIS/A_50mM_TRIS/50mA/TRIS_50mM_50mA_000159.tif", path "C:/Daten/pHGradienten/130403_Cy5_74mer_TRIS/130403_Cy5_74mer_TRIS/A_50mM_TRIS/50mA/TRIS_50mM_50mA_000160.tif", path "C:/Daten/pHGradienten/130403_Cy5_74mer_TRIS/130403_Cy5_74mer_TRIS/A_50mM_TRIS/50mA/TRIS_50mM_50mA_000161.tif", path "C:/Daten/pHGradienten/130403_Cy5_74mer_TRIS/130403_Cy5_74mer_TRIS/A_50mM_TRIS/50mA/TRIS_50mM_50mA_000162.tif", path "C:/Daten/pHGradienten/130403_Cy5_74mer_TRIS/130403_Cy5_74mer_TRIS/A_50mM_TRIS/50mA/TRIS_50mM_50mA_000163.tif", path "C:/Daten/pHGradienten/130403_Cy5_74mer_TRIS/130403_Cy5_74mer_TRIS/A_50mM_TRIS/50mA/TRIS_50mM_50mA_000164.tif", path "C:/Daten/pHGradienten/130403_Cy5_74mer_TRIS/130403_Cy5_74mer_TRIS/A_50mM_TRIS/50mA/TRIS_50mM_50mA_000165.tif", path "C:/Daten/pHGradienten/130403_Cy5_74mer_TRIS/130403_Cy5_74mer_TRIS/A_50mM_TRIS/50mA/TRIS_50mM_50mA_000166.tif", path "C:/Daten/pHGradienten/130403_Cy5_74mer_TRIS/130403_Cy5_74mer_TRIS/A_50mM_TRIS/50mA/TRIS_50mM_50mA_000167.tif", path "C:/Daten/pHGradienten/130403_Cy5_74mer_TRIS/130403_Cy5_74mer_TRIS/A_50mM_TRIS/50mA/TRIS_50mM_50mA_000168.tif", path "C:/Daten/pHGradienten/130403_Cy5_74mer_TRIS/130403_Cy5_74mer_TRIS/A_50mM_TRIS/50mA/TRIS_50mM_50mA_000169.tif", path "C:/Daten/pHGradienten/130403_Cy5_74mer_TRIS/130403_Cy5_74mer_TRIS/A_50mM_TRIS/50mA/TRIS_50mM_50mA_000170.tif", path "C:/Daten/pHGradienten/130403_Cy5_74mer_TRIS/130403_Cy5_74mer_TRIS/A_50mM_TRIS/50mA/TRIS_50mM_50mA_000171.tif", path "C:/Daten/pHGradienten/130403_Cy5_74mer_TRIS/130403_Cy5_74mer_TRIS/A_50mM_TRIS/50mA/TRIS_50mM_50mA_000172.tif", path "C:/Daten/pHGradienten/130403_Cy5_74mer_TRIS/130403_Cy5_74mer_TRIS/A_50mM_TRIS/50mA/TRIS_50mM_50mA_000173.tif", path "C:/Daten/pHGradienten/130403_Cy5_74mer_TRIS/130403_Cy5_74mer_TRIS/A_50mM_TRIS/50mA/TRIS_50mM_50mA_000174.tif", path "C:/Daten/pHGradienten/130403_Cy5_74mer_TRIS/130403_Cy5_74mer_TRIS/A_50mM_TRIS/50mA/TRIS_50mM_50mA_000175.tif", path "C:/Daten/pHGradienten/130403_Cy5_74mer_TRIS/130403_Cy5_74mer_TRIS/A_50mM_TRIS/50mA/TRIS_50mM_50mA_000176.tif", path "C:/Daten/pHGradienten/130403_Cy5_74mer_TRIS/130403_Cy5_74mer_TRIS/A_50mM_TRIS/50mA/TRIS_50mM_50mA_000177.tif", path "C:/Daten/pHGradienten/130403_Cy5_74mer_TRIS/130403_Cy5_74mer_TRIS/A_50mM_TRIS/50mA/TRIS_50mM_50mA_000178.tif", path "C:/Daten/pHGradienten/130403_Cy5_74mer_TRIS/130403_Cy5_74mer_TRIS/A_50mM_TRIS/50mA/TRIS_50mM_50mA_000179.tif", path "C:/Daten/pHGradienten/130403_Cy5_74mer_TRIS/130403_Cy5_74mer_TRIS/A_50mM_TRIS/50mA/TRIS_50mM_50mA_000180.tif", path "C:/Daten/pHGradienten/130403_Cy5_74mer_TRIS/130403_Cy5_74mer_TRIS/A_50mM_TRIS/50mA/TRIS_50mM_50mA_000181.tif", path "C:/Daten/pHGradienten/130403_Cy5_74mer_TRIS/130403_Cy5_74mer_TRIS/A_50mM_TRIS/50mA/TRIS_50mM_50mA_000182.tif", path "C:/Daten/pHGradienten/130403_Cy5_74mer_TRIS/130403_Cy5_74mer_TRIS/A_50mM_TRIS/50mA/TRIS_50mM_50mA_000183.tif", path "C:/Daten/pHGradienten/130403_Cy5_74mer_TRIS/130403_Cy5_74mer_TRIS/A_50mM_TRIS/50mA/TRIS_50mM_50mA_000184.tif", path "C:/Daten/pHGradienten/130403_Cy5_74mer_TRIS/130403_Cy5_74mer_TRIS/A_50mM_TRIS/50mA/TRIS_50mM_50mA_000185.tif", path "C:/Daten/pHGradienten/130403_Cy5_74mer_TRIS/130403_Cy5_74mer_TRIS/A_50mM_TRIS/50mA/TRIS_50mM_50mA_000186.tif", path "C:/Daten/pHGradienten/130403_Cy5_74mer_TRIS/130403_Cy5_74mer_TRIS/A_50mM_TRIS/50mA/TRIS_50mM_50mA_000187.tif", path "C:/Daten/pHGradienten/130403_Cy5_74mer_TRIS/130403_Cy5_74mer_TRIS/A_50mM_TRIS/50mA/TRIS_50mM_50mA_000188.tif", path "C:/Daten/pHGradienten/130403_Cy5_74mer_TRIS/130403_Cy5_74mer_TRIS/A_50mM_TRIS/50mA/TRIS_50mM_50mA_000189.tif", path "C:/Daten/pHGradienten/130403_Cy5_74mer_TRIS/130403_Cy5_74mer_TRIS/A_50mM_TRIS/50mA/TRIS_50mM_50mA_000190.tif", path "C:/Daten/pHGradienten/130403_Cy5_74mer_TRIS/130403_Cy5_74mer_TRIS/A_50mM_TRIS/50mA/TRIS_50mM_50mA_000191.tif", path "C:/Daten/pHGradienten/130403_Cy5_74mer_TRIS/130403_Cy5_74mer_TRIS/A_50mM_TRIS/50mA/TRIS_50mM_50mA_000192.tif", path "C:/Daten/pHGradienten/130403_Cy5_74mer_TRIS/130403_Cy5_74mer_TRIS/A_50mM_TRIS/50mA/TRIS_50mM_50mA_000193.tif", path "C:/Daten/pHGradienten/130403_Cy5_74mer_TRIS/130403_Cy5_74mer_TRIS/A_50mM_TRIS/50mA/TRIS_50mM_50mA_000194.tif", path "C:/Daten/pHGradienten/130403_Cy5_74mer_TRIS/130403_Cy5_74mer_TRIS/A_50mM_TRIS/50mA/TRIS_50mM_50mA_000195.tif", path "C:/Daten/pHGradienten/130403_Cy5_74mer_TRIS/130403_Cy5_74mer_TRIS/A_50mM_TRIS/50mA/TRIS_50mM_50mA_000196.tif", path "C:/Daten/pHGradienten/130403_Cy5_74mer_TRIS/130403_Cy5_74mer_TRIS/A_50mM_TRIS/50mA/TRIS_50mM_50mA_000197.tif", path "C:/Daten/pHGradienten/130403_Cy5_74mer_TRIS/130403_Cy5_74mer_TRIS/A_50mM_TRIS/50mA/TRIS_50mM_50mA_000198.tif", path "C:/Daten/pHGradienten/130403_Cy5_74mer_TRIS/130403_Cy5_74mer_TRIS/A_50mM_TRIS/50mA/TRIS_50mM_50mA_000199.tif", path "C:/Daten/pHGradienten/130403_Cy5_74mer_TRIS/130403_Cy5_74mer_TRIS/A_50mM_TRIS/50mA/TRIS_50mM_50mA_000200.tif", path "C:/Daten/pHGradienten/130403_Cy5_74mer_TRIS/130403_Cy5_74mer_TRIS/A_50mM_TRIS/50mA/TRIS_50mM_50mA_000201.tif", path "C:/Daten/pHGradienten/130403_Cy5_74mer_TRIS/130403_Cy5_74mer_TRIS/A_50mM_TRIS/50mA/TRIS_50mM_50mA_000202.tif", path "C:/Daten/pHGradienten/130403_Cy5_74mer_TRIS/130403_Cy5_74mer_TRIS/A_50mM_TRIS/50mA/TRIS_50mM_50mA_000203.tif", path "C:/Daten/pHGradienten/130403_Cy5_74mer_TRIS/130403_Cy5_74mer_TRIS/A_50mM_TRIS/50mA/TRIS_50mM_50mA_000204.tif", path "C:/Daten/pHGradienten/130403_Cy5_74mer_TRIS/130403_Cy5_74mer_TRIS/A_50mM_TRIS/50mA/TRIS_50mM_50mA_000205.tif", path "C:/Daten/pHGradienten/130403_Cy5_74mer_TRIS/130403_Cy5_74mer_TRIS/A_50mM_TRIS/50mA/TRIS_50mM_50mA_000206.tif", path "C:/Daten/pHGradienten/130403_Cy5_74mer_TRIS/130403_Cy5_74mer_TRIS/A_50mM_TRIS/50mA/TRIS_50mM_50mA_000207.tif", path "C:/Daten/pHGradienten/130403_Cy5_74mer_TRIS/130403_Cy5_74mer_TRIS/A_50mM_TRIS/50mA/TRIS_50mM_50mA_000208.tif", path "C:/Daten/pHGradienten/130403_Cy5_74mer_TRIS/130403_Cy5_74mer_TRIS/A_50mM_TRIS/50mA/TRIS_50mM_50mA_000209.tif", path "C:/Daten/pHGradienten/130403_Cy5_74mer_TRIS/130403_Cy5_74mer_TRIS/A_50mM_TRIS/50mA/TRIS_50mM_50mA_000210.tif", path "C:/Daten/pHGradienten/130403_Cy5_74mer_TRIS/130403_Cy5_74mer_TRIS/A_50mM_TRIS/50mA/TRIS_50mM_50mA_000211.tif", path "C:/Daten/pHGradienten/130403_Cy5_74mer_TRIS/130403_Cy5_74mer_TRIS/A_50mM_TRIS/50mA/TRIS_50mM_50mA_000212.tif", path "C:/Daten/pHGradienten/130403_Cy5_74mer_TRIS/130403_Cy5_74mer_TRIS/A_50mM_TRIS/50mA/TRIS_50mM_50mA_000213.tif", path "C:/Daten/pHGradienten/130403_Cy5_74mer_TRIS/130403_Cy5_74mer_TRIS/A_50mM_TRIS/50mA/TRIS_50mM_50mA_000214.tif", path "C:/Daten/pHGradienten/130403_Cy5_74mer_TRIS/130403_Cy5_74mer_TRIS/A_50mM_TRIS/50mA/TRIS_50mM_50mA_000215.tif", path "C:/Daten/pHGradienten/130403_Cy5_74mer_TRIS/130403_Cy5_74mer_TRIS/A_50mM_TRIS/50mA/TRIS_50mM_50mA_000216.tif", path "C:/Daten/pHGradienten/130403_Cy5_74mer_TRIS/130403_Cy5_74mer_TRIS/A_50mM_TRIS/50mA/TRIS_50mM_50mA_000217.tif", path "C:/Daten/pHGradienten/130403_Cy5_74mer_TRIS/130403_Cy5_74mer_TRIS/A_50mM_TRIS/50mA/TRIS_50mM_50mA_000218.tif", path "C:/Daten/pHGradienten/130403_Cy5_74mer_TRIS/130403_Cy5_74mer_TRIS/A_50mM_TRIS/50mA/TRIS_50mM_50mA_000219.tif", path "C:/Daten/pHGradienten/130403_Cy5_74mer_TRIS/130403_Cy5_74mer_TRIS/A_50mM_TRIS/50mA/TRIS_50mM_50mA_000220.tif", path "C:/Daten/pHGradienten/130403_Cy5_74mer_TRIS/130403_Cy5_74mer_TRIS/A_50mM_TRIS/50mA/TRIS_50mM_50mA_000221.tif", path "C:/Daten/pHGradienten/130403_Cy5_74mer_TRIS/130403_Cy5_74mer_TRIS/A_50mM_TRIS/50mA/TRIS_50mM_50mA_000222.tif", path "C:/Daten/pHGradienten/130403_Cy5_74mer_TRIS/130403_Cy5_74mer_TRIS/A_50mM_TRIS/50mA/TRIS_50mM_50mA_000223.tif", path "C:/Daten/pHGradienten/130403_Cy5_74mer_TRIS/130403_Cy5_74mer_TRIS/A_50mM_TRIS/50mA/TRIS_50mM_50mA_000224.tif", path "C:/Daten/pHGradienten/130403_Cy5_74mer_TRIS/130403_Cy5_74mer_TRIS/A_50mM_TRIS/50mA/TRIS_50mM_50mA_000225.tif", path "C:/Daten/pHGradienten/130403_Cy5_74mer_TRIS/130403_Cy5_74mer_TRIS/A_50mM_TRIS/50mA/TRIS_50mM_50mA_000226.tif", path "C:/Daten/pHGradienten/130403_Cy5_74mer_TRIS/130403_Cy5_74mer_TRIS/A_50mM_TRIS/50mA/TRIS_50mM_50mA_000227.tif", path "C:/Daten/pHGradienten/130403_Cy5_74mer_TRIS/130403_Cy5_74mer_TRIS/A_50mM_TRIS/50mA/TRIS_50mM_50mA_000228.tif", path "C:/Daten/pHGradienten/130403_Cy5_74mer_TRIS/130403_Cy5_74mer_TRIS/A_50mM_TRIS/50mA/TRIS_50mM_50mA_000229.tif", path "C:/Daten/pHGradienten/130403_Cy5_74mer_TRIS/130403_Cy5_74mer_TRIS/A_50mM_TRIS/50mA/TRIS_50mM_50mA_000230.tif", path "C:/Daten/pHGradienten/130403_Cy5_74mer_TRIS/130403_Cy5_74mer_TRIS/A_50mM_TRIS/50mA/TRIS_50mM_50mA_000231.tif", path "C:/Daten/pHGradienten/130403_Cy5_74mer_TRIS/130403_Cy5_74mer_TRIS/A_50mM_TRIS/50mA/TRIS_50mM_50mA_000232.tif", path "C:/Daten/pHGradienten/130403_Cy5_74mer_TRIS/130403_Cy5_74mer_TRIS/A_50mM_TRIS/50mA/TRIS_50mM_50mA_000233.tif", path "C:/Daten/pHGradienten/130403_Cy5_74mer_TRIS/130403_Cy5_74mer_TRIS/A_50mM_TRIS/50mA/TRIS_50mM_50mA_000234.tif", path "C:/Daten/pHGradienten/130403_Cy5_74mer_TRIS/130403_Cy5_74mer_TRIS/A_50mM_TRIS/50mA/TRIS_50mM_50mA_000235.tif", path "C:/Daten/pHGradienten/130403_Cy5_74mer_TRIS/130403_Cy5_74mer_TRIS/A_50mM_TRIS/50mA/TRIS_50mM_50mA_000236.tif", path "C:/Daten/pHGradienten/130403_Cy5_74mer_TRIS/130403_Cy5_74mer_TRIS/A_50mM_TRIS/50mA/TRIS_50mM_50mA_000237.tif", path "C:/Daten/pHGradienten/130403_Cy5_74mer_TRIS/130403_Cy5_74mer_TRIS/A_50mM_TRIS/50mA/TRIS_50mM_50mA_000238.tif", path "C:/Daten/pHGradienten/130403_Cy5_74mer_TRIS/130403_Cy5_74mer_TRIS/A_50mM_TRIS/50mA/TRIS_50mM_50mA_000239.tif", path "C:/Daten/pHGradienten/130403_Cy5_74mer_TRIS/130403_Cy5_74mer_TRIS/A_50mM_TRIS/50mA/TRIS_50mM_50mA_000240.tif", path "C:/Daten/pHGradienten/130403_Cy5_74mer_TRIS/130403_Cy5_74mer_TRIS/A_50mM_TRIS/50mA/TRIS_50mM_50mA_000241.tif", path "C:/Daten/pHGradienten/130403_Cy5_74mer_TRIS/130403_Cy5_74mer_TRIS/A_50mM_TRIS/50mA/TRIS_50mM_50mA_000242.tif", path "C:/Daten/pHGradienten/130403_Cy5_74mer_TRIS/130403_Cy5_74mer_TRIS/A_50mM_TRIS/50mA/TRIS_50mM_50mA_000243.tif", path "C:/Daten/pHGradienten/130403_Cy5_74mer_TRIS/130403_Cy5_74mer_TRIS/A_50mM_TRIS/50mA/TRIS_50mM_50mA_000244.tif", path "C:/Daten/pHGradienten/130403_Cy5_74mer_TRIS/130403_Cy5_74mer_TRIS/A_50mM_TRIS/50mA/TRIS_50mM_50mA_000245.tif", path "C:/Daten/pHGradienten/130403_Cy5_74mer_TRIS/130403_Cy5_74mer_TRIS/A_50mM_TRIS/50mA/TRIS_50mM_50mA_000246.tif", path "C:/Daten/pHGradienten/130403_Cy5_74mer_TRIS/130403_Cy5_74mer_TRIS/A_50mM_TRIS/50mA/TRIS_50mM_50mA_000247.tif", path "C:/Daten/pHGradienten/130403_Cy5_74mer_TRIS/130403_Cy5_74mer_TRIS/A_50mM_TRIS/50mA/TRIS_50mM_50mA_000248.tif", path "C:/Daten/pHGradienten/130403_Cy5_74mer_TRIS/130403_Cy5_74mer_TRIS/A_50mM_TRIS/50mA/TRIS_50mM_50mA_000249.tif", path "C:/Daten/pHGradienten/130403_Cy5_74mer_TRIS/130403_Cy5_74mer_TRIS/A_50mM_TRIS/50mA/TRIS_50mM_50mA_000250.tif", path "C:/Daten/pHGradienten/130403_Cy5_74mer_TRIS/130403_Cy5_74mer_TRIS/A_50mM_TRIS/50mA/TRIS_50mM_50mA_000251.tif", path "C:/Daten/pHGradienten/130403_Cy5_74mer_TRIS/130403_Cy5_74mer_TRIS/A_50mM_TRIS/50mA/TRIS_50mM_50mA_000252.tif", path "C:/Daten/pHGradienten/130403_Cy5_74mer_TRIS/130403_Cy5_74mer_TRIS/A_50mM_TRIS/50mA/TRIS_50mM_50mA_000253.tif", path "C:/Daten/pHGradienten/130403_Cy5_74mer_TRIS/130403_Cy5_74mer_TRIS/A_50mM_TRIS/50mA/TRIS_50mM_50mA_000254.tif", path "C:/Daten/pHGradienten/130403_Cy5_74mer_TRIS/130403_Cy5_74mer_TRIS/A_50mM_TRIS/50mA/TRIS_50mM_50mA_000255.tif", path "C:/Daten/pHGradienten/130403_Cy5_74mer_TRIS/130403_Cy5_74mer_TRIS/A_50mM_TRIS/50mA/TRIS_50mM_50mA_000256.tif", path "C:/Daten/pHGradienten/130403_Cy5_74mer_TRIS/130403_Cy5_74mer_TRIS/A_50mM_TRIS/50mA/TRIS_50mM_50mA_000257.tif", path "C:/Daten/pHGradienten/130403_Cy5_74mer_TRIS/130403_Cy5_74mer_TRIS/A_50mM_TRIS/50mA/TRIS_50mM_50mA_000258.tif", path "C:/Daten/pHGradienten/130403_Cy5_74mer_TRIS/130403_Cy5_74mer_TRIS/A_50mM_TRIS/50mA/TRIS_50mM_50mA_000259.tif", path "C:/Daten/pHGradienten/130403_Cy5_74mer_TRIS/130403_Cy5_74mer_TRIS/A_50mM_TRIS/50mA/TRIS_50mM_50mA_000260.tif", path "C:/Daten/pHGradienten/130403_Cy5_74mer_TRIS/130403_Cy5_74mer_TRIS/A_50mM_TRIS/50mA/TRIS_50mM_50mA_000261.tif", path "C:/Daten/pHGradienten/130403_Cy5_74mer_TRIS/130403_Cy5_74mer_TRIS/A_50mM_TRIS/50mA/TRIS_50mM_50mA_000262.tif", path "C:/Daten/pHGradienten/130403_Cy5_74mer_TRIS/130403_Cy5_74mer_TRIS/A_50mM_TRIS/50mA/TRIS_50mM_50mA_000263.tif", path "C:/Daten/pHGradienten/130403_Cy5_74mer_TRIS/130403_Cy5_74mer_TRIS/A_50mM_TRIS/50mA/TRIS_50mM_50mA_000264.tif", path "C:/Daten/pHGradienten/130403_Cy5_74mer_TRIS/130403_Cy5_74mer_TRIS/A_50mM_TRIS/50mA/TRIS_50mM_50mA_000265.tif", path "C:/Daten/pHGradienten/130403_Cy5_74mer_TRIS/130403_Cy5_74mer_TRIS/A_50mM_TRIS/50mA/TRIS_50mM_50mA_000266.tif", path "C:/Daten/pHGradienten/130403_Cy5_74mer_TRIS/130403_Cy5_74mer_TRIS/A_50mM_TRIS/50mA/TRIS_50mM_50mA_000267.tif", path "C:/Daten/pHGradienten/130403_Cy5_74mer_TRIS/130403_Cy5_74mer_TRIS/A_50mM_TRIS/50mA/TRIS_50mM_50mA_000268.tif", path "C:/Daten/pHGradienten/130403_Cy5_74mer_TRIS/130403_Cy5_74mer_TRIS/A_50mM_TRIS/50mA/TRIS_50mM_50mA_000269.tif", path "C:/Daten/pHGradienten/130403_Cy5_74mer_TRIS/130403_Cy5_74mer_TRIS/A_50mM_TRIS/50mA/TRIS_50mM_50mA_000270.tif", path "C:/Daten/pHGradienten/130403_Cy5_74mer_TRIS/130403_Cy5_74mer_TRIS/A_50mM_TRIS/50mA/TRIS_50mM_50mA_000271.tif", path "C:/Daten/pHGradienten/130403_Cy5_74mer_TRIS/130403_Cy5_74mer_TRIS/A_50mM_TRIS/50mA/TRIS_50mM_50mA_000272.tif", path "C:/Daten/pHGradienten/130403_Cy5_74mer_TRIS/130403_Cy5_74mer_TRIS/A_50mM_TRIS/50mA/TRIS_50mM_50mA_000273.tif", path "C:/Daten/pHGradienten/130403_Cy5_74mer_TRIS/130403_Cy5_74mer_TRIS/A_50mM_TRIS/50mA/TRIS_50mM_50mA_000274.tif", path "C:/Daten/pHGradienten/130403_Cy5_74mer_TRIS/130403_Cy5_74mer_TRIS/A_50mM_TRIS/50mA/TRIS_50mM_50mA_000275.tif", path "C:/Daten/pHGradienten/130403_Cy5_74mer_TRIS/130403_Cy5_74mer_TRIS/A_50mM_TRIS/50mA/TRIS_50mM_50mA_000276.tif", path "C:/Daten/pHGradienten/130403_Cy5_74mer_TRIS/130403_Cy5_74mer_TRIS/A_50mM_TRIS/50mA/TRIS_50mM_50mA_000277.tif", path "C:/Daten/pHGradienten/130403_Cy5_74mer_TRIS/130403_Cy5_74mer_TRIS/A_50mM_TRIS/50mA/TRIS_50mM_50mA_000278.tif", path "C:/Daten/pHGradienten/130403_Cy5_74mer_TRIS/130403_Cy5_74mer_TRIS/A_50mM_TRIS/50mA/TRIS_50mM_50mA_000279.tif", path "C:/Daten/pHGradienten/130403_Cy5_74mer_TRIS/130403_Cy5_74mer_TRIS/A_50mM_TRIS/50mA/TRIS_50mM_50mA_000280.tif", path "C:/Daten/pHGradienten/130403_Cy5_74mer_TRIS/130403_Cy5_74mer_TRIS/A_50mM_TRIS/50mA/TRIS_50mM_50mA_000281.tif", path "C:/Daten/pHGradienten/130403_Cy5_74mer_TRIS/130403_Cy5_74mer_TRIS/A_50mM_TRIS/50mA/TRIS_50mM_50mA_000282.tif", path "C:/Daten/pHGradienten/130403_Cy5_74mer_TRIS/130403_Cy5_74mer_TRIS/A_50mM_TRIS/50mA/TRIS_50mM_50mA_000283.tif", path "C:/Daten/pHGradienten/130403_Cy5_74mer_TRIS/130403_Cy5_74mer_TRIS/A_50mM_TRIS/50mA/TRIS_50mM_50mA_000284.tif", path "C:/Daten/pHGradienten/130403_Cy5_74mer_TRIS/130403_Cy5_74mer_TRIS/A_50mM_TRIS/50mA/TRIS_50mM_50mA_000285.tif", path "C:/Daten/pHGradienten/130403_Cy5_74mer_TRIS/130403_Cy5_74mer_TRIS/A_50mM_TRIS/50mA/TRIS_50mM_50mA_000286.tif", path "C:/Daten/pHGradienten/130403_Cy5_74mer_TRIS/130403_Cy5_74mer_TRIS/A_50mM_TRIS/50mA/TRIS_50mM_50mA_000287.tif", path "C:/Daten/pHGradienten/130403_Cy5_74mer_TRIS/130403_Cy5_74mer_TRIS/A_50mM_TRIS/50mA/TRIS_50mM_50mA_000288.tif", path "C:/Daten/pHGradienten/130403_Cy5_74mer_TRIS/130403_Cy5_74mer_TRIS/A_50mM_TRIS/50mA/TRIS_50mM_50mA_000289.tif", path "C:/Daten/pHGradienten/130403_Cy5_74mer_TRIS/130403_Cy5_74mer_TRIS/A_50mM_TRIS/50mA/TRIS_50mM_50mA_000290.tif", path "C:/Daten/pHGradienten/130403_Cy5_74mer_TRIS/130403_Cy5_74mer_TRIS/A_50mM_TRIS/50mA/TRIS_50mM_50mA_000291.tif", path "C:/Daten/pHGradienten/130403_Cy5_74mer_TRIS/130403_Cy5_74mer_TRIS/A_50mM_TRIS/50mA/TRIS_50mM_50mA_000292.tif", path "C:/Daten/pHGradienten/130403_Cy5_74mer_TRIS/130403_Cy5_74mer_TRIS/A_50mM_TRIS/50mA/TRIS_50mM_50mA_000293.tif", path "C:/Daten/pHGradienten/130403_Cy5_74mer_TRIS/130403_Cy5_74mer_TRIS/A_50mM_TRIS/50mA/TRIS_50mM_50mA_000294.tif", path "C:/Daten/pHGradienten/130403_Cy5_74mer_TRIS/130403_Cy5_74mer_TRIS/A_50mM_TRIS/50mA/TRIS_50mM_50mA_000295.tif", path "C:/Daten/pHGradienten/130403_Cy5_74mer_TRIS/130403_Cy5_74mer_TRIS/A_50mM_TRIS/50mA/TRIS_50mM_50mA_000296.tif", path "C:/Daten/pHGradienten/130403_Cy5_74mer_TRIS/130403_Cy5_74mer_TRIS/A_50mM_TRIS/50mA/TRIS_50mM_50mA_000297.tif", path "C:/Daten/pHGradienten/130403_Cy5_74mer_TRIS/130403_Cy5_74mer_TRIS/A_50mM_TRIS/50mA/TRIS_50mM_50mA_000298.tif", path "C:/Daten/pHGradienten/130403_Cy5_74mer_TRIS/130403_Cy5_74mer_TRIS/A_50mM_TRIS/50mA/TRIS_50mM_50mA_000299.tif", path "C:/Daten/pHGradienten/130403_Cy5_74mer_TRIS/130403_Cy5_74mer_TRIS/A_50mM_TRIS/50mA/TRIS_50mM_50mA_000300.tif", path "C:/Daten/pHGradienten/130403_Cy5_74mer_TRIS/130403_Cy5_74mer_TRIS/A_50mM_TRIS/50mA/TRIS_50mM_50mA_000301.tif", path "C:/Daten/pHGradienten/130403_Cy5_74mer_TRIS/130403_Cy5_74mer_TRIS/A_50mM_TRIS/50mA/TRIS_50mM_50mA_000302.tif", path "C:/Daten/pHGradienten/130403_Cy5_74mer_TRIS/130403_Cy5_74mer_TRIS/A_50mM_TRIS/50mA/TRIS_50mM_50mA_000303.tif", path "C:/Daten/pHGradienten/130403_Cy5_74mer_TRIS/130403_Cy5_74mer_TRIS/A_50mM_TRIS/50mA/TRIS_50mM_50mA_000304.tif", path "C:/Daten/pHGradienten/130403_Cy5_74mer_TRIS/130403_Cy5_74mer_TRIS/A_50mM_TRIS/50mA/TRIS_50mM_50mA_000305.tif", path "C:/Daten/pHGradienten/130403_Cy5_74mer_TRIS/130403_Cy5_74mer_TRIS/A_50mM_TRIS/50mA/TRIS_50mM_50mA_000306.tif", path "C:/Daten/pHGradienten/130403_Cy5_74mer_TRIS/130403_Cy5_74mer_TRIS/A_50mM_TRIS/50mA/TRIS_50mM_50mA_000307.tif", path "C:/Daten/pHGradienten/130403_Cy5_74mer_TRIS/130403_Cy5_74mer_TRIS/A_50mM_TRIS/50mA/TRIS_50mM_50mA_000308.tif", path "C:/Daten/pHGradienten/130403_Cy5_74mer_TRIS/130403_Cy5_74mer_TRIS/A_50mM_TRIS/50mA/TRIS_50mM_50mA_000309.tif", path "C:/Daten/pHGradienten/130403_Cy5_74mer_TRIS/130403_Cy5_74mer_TRIS/A_50mM_TRIS/50mA/TRIS_50mM_50mA_000310.tif", path "C:/Daten/pHGradienten/130403_Cy5_74mer_TRIS/130403_Cy5_74mer_TRIS/A_50mM_TRIS/50mA/TRIS_50mM_50mA_000311.tif", path "C:/Daten/pHGradienten/130403_Cy5_74mer_TRIS/130403_Cy5_74mer_TRIS/A_50mM_TRIS/50mA/TRIS_50mM_50mA_000312.tif", path "C:/Daten/pHGradienten/130403_Cy5_74mer_TRIS/130403_Cy5_74mer_TRIS/A_50mM_TRIS/50mA/TRIS_50mM_50mA_000313.tif", path "C:/Daten/pHGradienten/130403_Cy5_74mer_TRIS/130403_Cy5_74mer_TRIS/A_50mM_TRIS/50mA/TRIS_50mM_50mA_000314.tif", path "C:/Daten/pHGradienten/130403_Cy5_74mer_TRIS/130403_Cy5_74mer_TRIS/A_50mM_TRIS/50mA/TRIS_50mM_50mA_000315.tif", path "C:/Daten/pHGradienten/130403_Cy5_74mer_TRIS/130403_Cy5_74mer_TRIS/A_50mM_TRIS/50mA/TRIS_50mM_50mA_000316.tif", path "C:/Daten/pHGradienten/130403_Cy5_74mer_TRIS/130403_Cy5_74mer_TRIS/A_50mM_TRIS/50mA/TRIS_50mM_50mA_000317.tif", path "C:/Daten/pHGradienten/130403_Cy5_74mer_TRIS/130403_Cy5_74mer_TRIS/A_50mM_TRIS/50mA/TRIS_50mM_50mA_000318.tif", path "C:/Daten/pHGradienten/130403_Cy5_74mer_TRIS/130403_Cy5_74mer_TRIS/A_50mM_TRIS/50mA/TRIS_50mM_50mA_000319.tif", path "C:/Daten/pHGradienten/130403_Cy5_74mer_TRIS/130403_Cy5_74mer_TRIS/A_50mM_TRIS/50mA/TRIS_50mM_50mA_000320.tif", path "C:/Daten/pHGradienten/130403_Cy5_74mer_TRIS/130403_Cy5_74mer_TRIS/A_50mM_TRIS/50mA/TRIS_50mM_50mA_000321.tif", path "C:/Daten/pHGradienten/130403_Cy5_74mer_TRIS/130403_Cy5_74mer_TRIS/A_50mM_TRIS/50mA/TRIS_50mM_50mA_000322.tif", path "C:/Daten/pHGradienten/130403_Cy5_74mer_TRIS/130403_Cy5_74mer_TRIS/A_50mM_TRIS/50mA/TRIS_50mM_50mA_000323.tif", path "C:/Daten/pHGradienten/130403_Cy5_74mer_TRIS/130403_Cy5_74mer_TRIS/A_50mM_TRIS/50mA/TRIS_50mM_50mA_000324.tif", path "C:/Daten/pHGradienten/130403_Cy5_74mer_TRIS/130403_Cy5_74mer_TRIS/A_50mM_TRIS/50mA/TRIS_50mM_50mA_000325.tif", path "C:/Daten/pHGradienten/130403_Cy5_74mer_TRIS/130403_Cy5_74mer_TRIS/A_50mM_TRIS/50mA/TRIS_50mM_50mA_000326.tif", path "C:/Daten/pHGradienten/130403_Cy5_74mer_TRIS/130403_Cy5_74mer_TRIS/A_50mM_TRIS/50mA/TRIS_50mM_50mA_000327.tif", path "C:/Daten/pHGradienten/130403_Cy5_74mer_TRIS/130403_Cy5_74mer_TRIS/A_50mM_TRIS/50mA/TRIS_50mM_50mA_000328.tif", path "C:/Daten/pHGradienten/130403_Cy5_74mer_TRIS/130403_Cy5_74mer_TRIS/A_50mM_TRIS/50mA/TRIS_50mM_50mA_000329.tif", path "C:/Daten/pHGradienten/130403_Cy5_74mer_TRIS/130403_Cy5_74mer_TRIS/A_50mM_TRIS/50mA/TRIS_50mM_50mA_000330.tif", path "C:/Daten/pHGradienten/130403_Cy5_74mer_TRIS/130403_Cy5_74mer_TRIS/A_50mM_TRIS/50mA/TRIS_50mM_50mA_000331.tif", path "C:/Daten/pHGradienten/130403_Cy5_74mer_TRIS/130403_Cy5_74mer_TRIS/A_50mM_TRIS/50mA/TRIS_50mM_50mA_000332.tif", path "C:/Daten/pHGradienten/130403_Cy5_74mer_TRIS/130403_Cy5_74mer_TRIS/A_50mM_TRIS/50mA/TRIS_50mM_50mA_000333.tif", path "C:/Daten/pHGradienten/130403_Cy5_74mer_TRIS/130403_Cy5_74mer_TRIS/A_50mM_TRIS/50mA/TRIS_50mM_50mA_000334.tif", path "C:/Daten/pHGradienten/130403_Cy5_74mer_TRIS/130403_Cy5_74mer_TRIS/A_50mM_TRIS/50mA/TRIS_50mM_50mA_000335.tif", path "C:/Daten/pHGradienten/130403_Cy5_74mer_TRIS/130403_Cy5_74mer_TRIS/A_50mM_TRIS/50mA/TRIS_50mM_50mA_000336.tif", path "C:/Daten/pHGradienten/130403_Cy5_74mer_TRIS/130403_Cy5_74mer_TRIS/A_50mM_TRIS/50mA/TRIS_50mM_50mA_000337.tif", path "C:/Daten/pHGradienten/130403_Cy5_74mer_TRIS/130403_Cy5_74mer_TRIS/A_50mM_TRIS/50mA/TRIS_50mM_50mA_000338.tif", path "C:/Daten/pHGradienten/130403_Cy5_74mer_TRIS/130403_Cy5_74mer_TRIS/A_50mM_TRIS/50mA/TRIS_50mM_50mA_000339.tif", path "C:/Daten/pHGradienten/130403_Cy5_74mer_TRIS/130403_Cy5_74mer_TRIS/A_50mM_TRIS/50mA/TRIS_50mM_50mA_000340.tif", path "C:/Daten/pHGradienten/130403_Cy5_74mer_TRIS/130403_Cy5_74mer_TRIS/A_50mM_TRIS/50mA/TRIS_50mM_50mA_000341.tif", path "C:/Daten/pHGradienten/130403_Cy5_74mer_TRIS/130403_Cy5_74mer_TRIS/A_50mM_TRIS/50mA/TRIS_50mM_50mA_000342.tif", path "C:/Daten/pHGradienten/130403_Cy5_74mer_TRIS/130403_Cy5_74mer_TRIS/A_50mM_TRIS/50mA/TRIS_50mM_50mA_000343.tif", path "C:/Daten/pHGradienten/130403_Cy5_74mer_TRIS/130403_Cy5_74mer_TRIS/A_50mM_TRIS/50mA/TRIS_50mM_50mA_000344.tif", path "C:/Daten/pHGradienten/130403_Cy5_74mer_TRIS/130403_Cy5_74mer_TRIS/A_50mM_TRIS/50mA/TRIS_50mM_50mA_000345.tif", path "C:/Daten/pHGradienten/130403_Cy5_74mer_TRIS/130403_Cy5_74mer_TRIS/A_50mM_TRIS/50mA/TRIS_50mM_50mA_000346.tif", path "C:/Daten/pHGradienten/130403_Cy5_74mer_TRIS/130403_Cy5_74mer_TRIS/A_50mM_TRIS/50mA/TRIS_50mM_50mA_000347.tif", path "C:/Daten/pHGradienten/130403_Cy5_74mer_TRIS/130403_Cy5_74mer_TRIS/A_50mM_TRIS/50mA/TRIS_50mM_50mA_000348.tif", path "C:/Daten/pHGradienten/130403_Cy5_74mer_TRIS/130403_Cy5_74mer_TRIS/A_50mM_TRIS/50mA/TRIS_50mM_50mA_000349.tif", path "C:/Daten/pHGradienten/130403_Cy5_74mer_TRIS/130403_Cy5_74mer_TRIS/A_50mM_TRIS/50mA/TRIS_50mM_50mA_000350.tif", path "C:/Daten/pHGradienten/130403_Cy5_74mer_TRIS/130403_Cy5_74mer_TRIS/A_50mM_TRIS/50mA/TRIS_50mM_50mA_000351.tif", path "C:/Daten/pHGradienten/130403_Cy5_74mer_TRIS/130403_Cy5_74mer_TRIS/A_50mM_TRIS/50mA/TRIS_50mM_50mA_000352.tif", path "C:/Daten/pHGradienten/130403_Cy5_74mer_TRIS/130403_Cy5_74mer_TRIS/A_50mM_TRIS/50mA/TRIS_50mM_50mA_000353.tif", path "C:/Daten/pHGradienten/130403_Cy5_74mer_TRIS/130403_Cy5_74mer_TRIS/A_50mM_TRIS/50mA/TRIS_50mM_50mA_000354.tif", path "C:/Daten/pHGradienten/130403_Cy5_74mer_TRIS/130403_Cy5_74mer_TRIS/A_50mM_TRIS/50mA/TRIS_50mM_50mA_000355.tif", path "C:/Daten/pHGradienten/130403_Cy5_74mer_TRIS/130403_Cy5_74mer_TRIS/A_50mM_TRIS/50mA/TRIS_50mM_50mA_000356.tif", path "C:/Daten/pHGradienten/130403_Cy5_74mer_TRIS/130403_Cy5_74mer_TRIS/A_50mM_TRIS/50mA/TRIS_50mM_50mA_000357.tif", path "C:/Daten/pHGradienten/130403_Cy5_74mer_TRIS/130403_Cy5_74mer_TRIS/A_50mM_TRIS/50mA/TRIS_50mM_50mA_000358.tif", path "C:/Daten/pHGradienten/130403_Cy5_74mer_TRIS/130403_Cy5_74mer_TRIS/A_50mM_TRIS/50mA/TRIS_50mM_50mA_000359.tif", path "C:/Daten/pHGradienten/130403_Cy5_74mer_TRIS/130403_Cy5_74mer_TRIS/A_50mM_TRIS/50mA/TRIS_50mM_50mA_000360.tif", path "C:/Daten/pHGradienten/130403_Cy5_74mer_TRIS/130403_Cy5_74mer_TRIS/A_50mM_TRIS/50mA/TRIS_50mM_50mA_000361.tif", path "C:/Daten/pHGradienten/130403_Cy5_74mer_TRIS/130403_Cy5_74mer_TRIS/A_50mM_TRIS/50mA/TRIS_50mM_50mA_000362.tif", path "C:/Daten/pHGradienten/130403_Cy5_74mer_TRIS/130403_Cy5_74mer_TRIS/A_50mM_TRIS/50mA/TRIS_50mM_50mA_000363.tif", path "C:/Daten/pHGradienten/130403_Cy5_74mer_TRIS/130403_Cy5_74mer_TRIS/A_50mM_TRIS/50mA/TRIS_50mM_50mA_000364.tif", path "C:/Daten/pHGradienten/130403_Cy5_74mer_TRIS/130403_Cy5_74mer_TRIS/A_50mM_TRIS/50mA/TRIS_50mM_50mA_000365.tif", path "C:/Daten/pHGradienten/130403_Cy5_74mer_TRIS/130403_Cy5_74mer_TRIS/A_50mM_TRIS/50mA/TRIS_50mM_50mA_000366.tif", path "C:/Daten/pHGradienten/130403_Cy5_74mer_TRIS/130403_Cy5_74mer_TRIS/A_50mM_TRIS/50mA/TRIS_50mM_50mA_000367.tif", path "C:/Daten/pHGradienten/130403_Cy5_74mer_TRIS/130403_Cy5_74mer_TRIS/A_50mM_TRIS/50mA/TRIS_50mM_50mA_000368.tif", path "C:/Daten/pHGradienten/130403_Cy5_74mer_TRIS/130403_Cy5_74mer_TRIS/A_50mM_TRIS/50mA/TRIS_50mM_50mA_000369.tif", path "C:/Daten/pHGradienten/130403_Cy5_74mer_TRIS/130403_Cy5_74mer_TRIS/A_50mM_TRIS/50mA/TRIS_50mM_50mA_000370.tif", path "C:/Daten/pHGradienten/130403_Cy5_74mer_TRIS/130403_Cy5_74mer_TRIS/A_50mM_TRIS/50mA/TRIS_50mM_50mA_000371.tif", path "C:/Daten/pHGradienten/130403_Cy5_74mer_TRIS/130403_Cy5_74mer_TRIS/A_50mM_TRIS/50mA/TRIS_50mM_50mA_000372.tif", path "C:/Daten/pHGradienten/130403_Cy5_74mer_TRIS/130403_Cy5_74mer_TRIS/A_50mM_TRIS/50mA/TRIS_50mM_50mA_000373.tif", path "C:/Daten/pHGradienten/130403_Cy5_74mer_TRIS/130403_Cy5_74mer_TRIS/A_50mM_TRIS/50mA/TRIS_50mM_50mA_000374.tif", path "C:/Daten/pHGradienten/130403_Cy5_74mer_TRIS/130403_Cy5_74mer_TRIS/A_50mM_TRIS/50mA/TRIS_50mM_50mA_000375.tif", path "C:/Daten/pHGradienten/130403_Cy5_74mer_TRIS/130403_Cy5_74mer_TRIS/A_50mM_TRIS/50mA/TRIS_50mM_50mA_000376.tif", path "C:/Daten/pHGradienten/130403_Cy5_74mer_TRIS/130403_Cy5_74mer_TRIS/A_50mM_TRIS/50mA/TRIS_50mM_50mA_000377.tif", path "C:/Daten/pHGradienten/130403_Cy5_74mer_TRIS/130403_Cy5_74mer_TRIS/A_50mM_TRIS/50mA/TRIS_50mM_50mA_000378.tif", path "C:/Daten/pHGradienten/130403_Cy5_74mer_TRIS/130403_Cy5_74mer_TRIS/A_50mM_TRIS/50mA/TRIS_50mM_50mA_000379.tif", path "C:/Daten/pHGradienten/130403_Cy5_74mer_TRIS/130403_Cy5_74mer_TRIS/A_50mM_TRIS/50mA/TRIS_50mM_50mA_000380.tif", path "C:/Daten/pHGradienten/130403_Cy5_74mer_TRIS/130403_Cy5_74mer_TRIS/A_50mM_TRIS/50mA/TRIS_50mM_50mA_000381.tif", path "C:/Daten/pHGradienten/130403_Cy5_74mer_TRIS/130403_Cy5_74mer_TRIS/A_50mM_TRIS/50mA/TRIS_50mM_50mA_000382.tif", path "C:/Daten/pHGradienten/130403_Cy5_74mer_TRIS/130403_Cy5_74mer_TRIS/A_50mM_TRIS/50mA/TRIS_50mM_50mA_000383.tif", path "C:/Daten/pHGradienten/130403_Cy5_74mer_TRIS/130403_Cy5_74mer_TRIS/A_50mM_TRIS/50mA/TRIS_50mM_50mA_000384.tif", path "C:/Daten/pHGradienten/130403_Cy5_74mer_TRIS/130403_Cy5_74mer_TRIS/A_50mM_TRIS/50mA/TRIS_50mM_50mA_000385.tif", path "C:/Daten/pHGradienten/130403_Cy5_74mer_TRIS/130403_Cy5_74mer_TRIS/A_50mM_TRIS/50mA/TRIS_50mM_50mA_000386.tif", path "C:/Daten/pHGradienten/130403_Cy5_74mer_TRIS/130403_Cy5_74mer_TRIS/A_50mM_TRIS/50mA/TRIS_50mM_50mA_000387.tif", path "C:/Daten/pHGradienten/130403_Cy5_74mer_TRIS/130403_Cy5_74mer_TRIS/A_50mM_TRIS/50mA/TRIS_50mM_50mA_000388.tif", path "C:/Daten/pHGradienten/130403_Cy5_74mer_TRIS/130403_Cy5_74mer_TRIS/A_50mM_TRIS/50mA/TRIS_50mM_50mA_000389.tif", path "C:/Daten/pHGradienten/130403_Cy5_74mer_TRIS/130403_Cy5_74mer_TRIS/A_50mM_TRIS/50mA/TRIS_50mM_50mA_000390.tif", path "C:/Daten/pHGradienten/130403_Cy5_74mer_TRIS/130403_Cy5_74mer_TRIS/A_50mM_TRIS/50mA/TRIS_50mM_50mA_000391.tif", path "C:/Daten/pHGradienten/130403_Cy5_74mer_TRIS/130403_Cy5_74mer_TRIS/A_50mM_TRIS/50mA/TRIS_50mM_50mA_000392.tif", path "C:/Daten/pHGradienten/130403_Cy5_74mer_TRIS/130403_Cy5_74mer_TRIS/A_50mM_TRIS/50mA/TRIS_50mM_50mA_000393.tif", path "C:/Daten/pHGradienten/130403_Cy5_74mer_TRIS/130403_Cy5_74mer_TRIS/A_50mM_TRIS/50mA/TRIS_50mM_50mA_000394.tif", path "C:/Daten/pHGradienten/130403_Cy5_74mer_TRIS/130403_Cy5_74mer_TRIS/A_50mM_TRIS/50mA/TRIS_50mM_50mA_000395.tif", path "C:/Daten/pHGradienten/130403_Cy5_74mer_TRIS/130403_Cy5_74mer_TRIS/A_50mM_TRIS/50mA/TRIS_50mM_50mA_000396.tif", path "C:/Daten/pHGradienten/130403_Cy5_74mer_TRIS/130403_Cy5_74mer_TRIS/A_50mM_TRIS/50mA/TRIS_50mM_50mA_000397.tif", path "C:/Daten/pHGradienten/130403_Cy5_74mer_TRIS/130403_Cy5_74mer_TRIS/A_50mM_TRIS/50mA/TRIS_50mM_50mA_000398.tif", path "C:/Daten/pHGradienten/130403_Cy5_74mer_TRIS/130403_Cy5_74mer_TRIS/A_50mM_TRIS/50mA/TRIS_50mM_50mA_000399.tif"], 7 "Background Offset":dbl, 8 "Cursor Cold1":dbl, 9 "Pixel Width [um/pixel]":dbl, 11 "Constant Background":dbl, 12 "Cursor Cold2":dbl, 13 "Binning":dbl, 14 "Cursor Hot1":dbl, 15 "Frame Time [s]":dbl, 16 "Cursor Hot2":dbl, 17 "Radial Resolution [pixel]":dbl) -> (20 "Hot Image":dbl[][](graph), 21 "Cold Image":dbl[][](graph), 23 "Hot/Cold":dbl[][](graph), 24 "X Projection":cluster{"Radius [um]":dbl[], "X-Average":dbl[]}(graph)={"Radius [um]"=[0.0, 12.9, 25.8, 38.7, 51.6, 64.5, 77.4, 90.3, 103.2, 116.10000000000001, 129.0, 141.9, 154.8, 167.70000000000002, 180.6, 193.5, 206.4, 219.3, 232.20000000000002, 245.1, 258.0, 270.90000000000003, 283.8, 296.7, 309.6, 322.5, 335.40000000000003], "X-Average"=[1.4112024251856488, 1.424926142625863, 1.4386176390234398, 1.444032817524326, 1.4425737257534479, 1.4239561945341481, 1.3949341654478993, 1.3661249397492634, 1.3382009359546228, 1.1864769982965713, 1.167152521599448, 1.1502392299709245, 1.133685190954566, 1.115322756815215, 1.0964568586521697, 1.0826863746950983, 1.0729876360478616]}, 25 "Y Projection":cluster{"Radius [um]":dbl[], "Y-Average":dbl[]}(graph)={"Radius [um]"=[0.0, 12.9, 25.8, 38.7, 51.6, 64.5, 77.4, 90.3, 103.2, 116.10000000000001, 129.0, 141.9, 154.8, 167.70000000000002, 180.6, 193.5, 206.4, 219.3, 232.20000000000002, 245.1, 258.0, 270.90000000000003, 283.8, 296.7, 309.6, 322.5, 335.40000000000003], "Y-Average"=[1.4112024251856488, 1.430663577211167, 1.481518832901356, 1.5348619479772767, 1.943330474160886, 1.9865101576139728, 1.8481972128370234, 1.7187536534015067, 1.636542946962924, 1.5571836581625942, 1.4398262418692351, 1.3025224024008983, 1.177310100194863, 1.0968282528155306, 1.0560824708604195, 1.0388818479949755, 1.0330012211788613, 1.0309133884891961, 1.0286453977828098, 1.028911824319958, 1.0284634631141085]}, 27 "Radial Average":T2(graph)={"Radius [um]"=[0.0, 12.9, 25.8, 38.7, 51.6, 64.5, 77.4, 90.3, 103.2, 116.10000000000001, 129.0, 141.9, 154.8, 167.70000000000002, 180.6, 193.5, 206.4, 219.3, 232.20000000000002, 245.1, 258.0, 270.90000000000003, 283.8, 296.7, 309.6, 322.5, 335.40000000000003], "Radial Average"=[1.4116794866580213, 1.4286286477793237, 1.462534494475321, 1.4924812794304163, 1.5627243682345884, 1.6072999892676256, 1.5872510962172341, 1.559811776121575, 1.5395965065434625, 1.5155166271077316, 1.4478604536943493, 1.3699343662317698, 1.2988180525975654, 1.2372326226316148, 1.1875961673215087, 1.150322754004717, 1.1257013618247929, 1.114061034221512, 1.094862455390781, 1.077694717135008, 1.0662476131304066, 1.0727644146422628, 1.0769216263834325, 1.0613000313352163, 1.0458047725299782, 1.0389359177801656, 1.0368515451091813]})   [LabVIEW 2010]
panel:
  in  "Substract \nBackground \nImages":T1(ring)
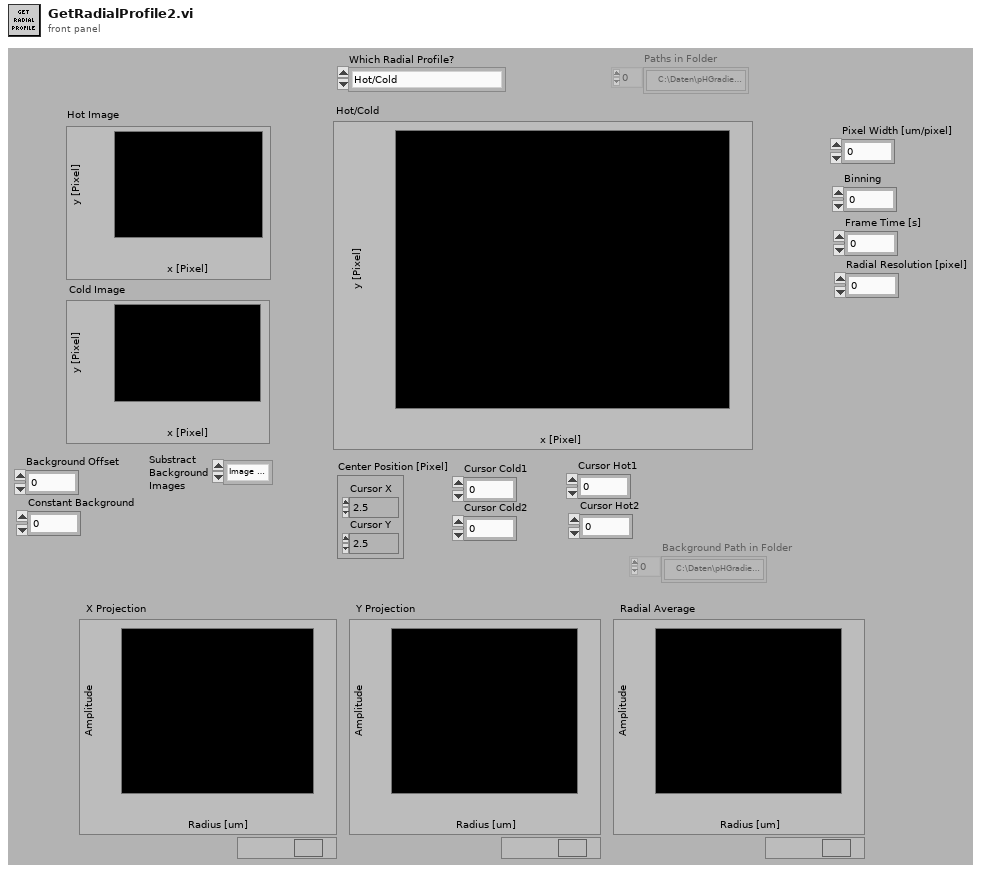
[diagram p1: front panel]
types:
  T1 = enum16{"Image by Image", "Single Image", "Constant Value"}
  T2 = cluster{"Radius [um]":dbl[], "Radial Average":dbl[]}
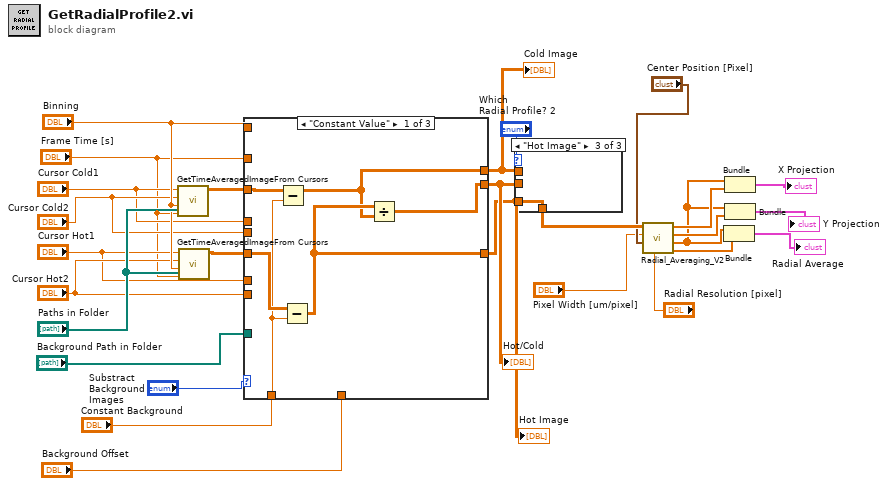
[diagram p0: block diagram]
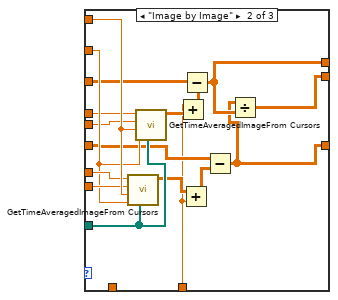
[diagram p2: hidden frame]
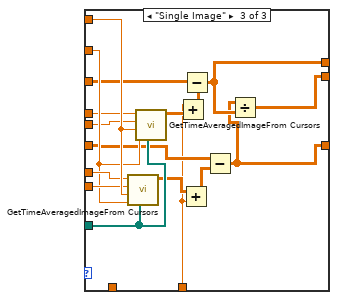
[diagram p3: hidden frame]
diagram:
  n1 = call "GetTimeAveragedImageFrom Cursors.vi"("Paths in Folder"="Paths in Folder", "Frame Time [s]"="Frame Time [s]", "Binning"="Binning", "Cursor 2"="Cursor Cold2", "Cursor 1"="Cursor Cold1") -> ("Averaged Image"=w7:dbl[][])  [unwired: 6 in]
  n2 = call "GetTimeAveragedImageFrom Cursors.vi"("Paths in Folder"="Paths in Folder", "Frame Time [s]"="Frame Time [s]", "Binning"="Binning", "Cursor 2"="Cursor Hot2", "Cursor 1"="Cursor Hot1") -> ("Averaged Image"=w15:dbl[][])  [unwired: 6 in]
  n3 = case shown="\"Constant Value\"" "Substract \nBackground \nImages" {
    tunnel: [w33 w51 w68] -> w3
    tunnel: w15 -> [w34 w42 w59]
    tunnel: "Binning" -> [_ w50 w67]
    tunnel: "Cursor Hot2" -> [_ w49 w66]
    tunnel: "Cursor Hot1" -> [_ w48 w65]
    tunnel: "Cursor Cold2" -> [_ w43 w60]
    tunnel: "Cursor Cold1" -> [_ w44 w61]
    tunnel: "Frame Time [s]" -> [_ w45 w62]
    tunnel: "Background Path in Folder" -> [_ w47 w64]
    tunnel: [w31 w39 w56] -> w2
    tunnel: w7 -> [w32 w41 w58]
    tunnel: [w30 w40 w57] -> w4
    tunnel: "Background Offset" -> [_ w35 w52]
    tunnel: "Constant Background" -> [w29 _ _]
    frame "Constant Value" {
      n4 = Subtract(x=w32, y=w29) -> (x-y=w30:dbl[][])
      n5 = Subtract(x=w34, y=w29) -> (x-y=w31:dbl[][])
      n6 = Divide(x=w31, y=w30) -> (x/y=w33:dbl[][])
    }
    frame "Image by Image" {
      n7 = call "GetTimeAveragedImageFrom Cursors.vi"("Paths in Folder"=w47, "Frame Time [s]"=w45, "Binning"=w50, "Cursor 2"=w49, "Cursor 1"=w48) -> ("Averaged Image"=w37:dbl[][])  [unwired: 6 in]
      n8 = call "GetTimeAveragedImageFrom Cursors.vi"("Paths in Folder"=w47, "Frame Time [s]"=w45, "Binning"=w50, "Cursor 2"=w43, "Cursor 1"=w44) -> ("Averaged Image"=w46:dbl[][])  [unwired: 6 in]
      n9 = Add(x=w35, y=w46) -> (x+y=w36:dbl[][])
      n10 = Add(x=w37, y=w35) -> (x+y=w38:dbl[][])
      n11 = Subtract(x=w41, y=w36) -> (x-y=w40:dbl[][])
      n12 = Subtract(x=w42, y=w38) -> (x-y=w39:dbl[][])
      n13 = Divide(x=w39, y=w40) -> (x/y=w51:dbl[][])
    }
    frame "Single Image" {
      n14 = call "GetTimeAveragedImageFrom Cursors.vi"("Paths in Folder"=w64, "Frame Time [s]"=w62, "Binning"=w67, "Cursor 2"=w66, "Cursor 1"=w65) -> ("Averaged Image"=w54:dbl[][])  [unwired: 6 in]
      n15 = call "GetTimeAveragedImageFrom Cursors.vi"("Paths in Folder"=w64, "Frame Time [s]"=w62, "Binning"=w67, "Cursor 2"=w60, "Cursor 1"=w61) -> ("Averaged Image"=w63:dbl[][])  [unwired: 6 in]
      n16 = Add(x=w52, y=w63) -> (x+y=w53:dbl[][])
      n17 = Add(x=w54, y=w52) -> (x+y=w55:dbl[][])
      n18 = Subtract(x=w58, y=w53) -> (x-y=w57:dbl[][])
      n19 = Subtract(x=w59, y=w55) -> (x-y=w56:dbl[][])
      n20 = Divide(x=w56, y=w57) -> (x/y=w68:dbl[][])
    }
  }
  "Cold Image" <- w4
  "Hot/Cold" <- w3
  "Hot Image" <- w2
  n21 = case shown="\"Hot Image\"" "Which \nRadial Profile? 2" {
    tunnel: w3 -> [_ w70 _]
    tunnel: w2 -> [_ _ w71]
    tunnel: w4 -> [w69 _ _]
    tunnel: [w69 w70 w71] -> w24
    frame "Cold Image", Default {
    }
    frame "Hot/Cold" {
    }
    frame "Hot Image" {
    }
  }
  n22 = call "Radial_Averaging_V2.vi"("Radial Resolution [pixel]"="Radial Resolution [pixel]", "Center Position [Pixel]"="Center Position [Pixel]", "Pixel Width [um/pixel]"="Pixel Width [um/pixel]", "Image"=w24) -> ("Radial Average"=w26:dbl[], "Radius [um]"=w25:dbl[], "Y-Average"=w28:dbl[], "X-Average"=w27:dbl[])  [unwired: 4 in]
  n23 = Bundle("Radius [um]"=w25, "Radial Average"=w26) -> (→"Radial Average":T2)  [unwired: 1 in]
  n24 = Bundle("Radius [um]"=w25, "X-Average"=w27) -> (→"X Projection":cluster{"Radius [um]":dbl[], "X-Average":dbl[]})  [unwired: 1 in]
  n25 = Bundle("Radius [um]"=w25, "Y-Average"=w28) -> (→"Y Projection":cluster{"Radius [um]":dbl[], "Y-Average":dbl[]})  [unwired: 1 in]
